vi "main 1.16 testing LR.vi"() -> ()   [LabVIEW 2015]
uses:
  subvi/PHOIBOS/DEFINITIONS/DEF_dev_state.ctl
  subvi/PHOIBOS/DEFINITIONS/DEF_dev_type.ctl
  <vilib>/Analysis/_algsub.llb/Real Vector Norm.vi
  <vilib>/Analysis/1siggen.llb/Ramp Pattern by Samples.vi
  <vilib>/DAQmx/create/channels.llb/DAQmx Create Channel (DI-Digital Input).vi
  <userlib>/caLab/Private/Put_DBL_PV.vi
  <vilib>/Utility/file.llb/Write Delimited Spreadsheet (string).vi
  <vilib>/Utility/file.llb/Read Delimited Spreadsheet (string).vi
  <vilib>/Utility/file.llb/Write Delimited Spreadsheet (DBL).vi
  <userlib>/caLab/Private/Get_PV.vi
  subvi/Newport ESP301/Newport ESP301.lvlib
  subvi/sp_manip.llb/sp_manip_lib.lvlib
  subvi/sp_manip.llb/tcp_gateway.lvlib
  <vilib>/Analysis/NI_AALBase.lvlib
  <vilib>/Analysis/NI_AALPro.lvlib
  subvi/ZaberTSeries/ZaberTSeries.lvlib
panel:
  out "Pics L":i32=200
  out "Waveform Chart":dbl(graph)
  out "G2 X":cluster{dbl[], "Ramp Pattern":dbl[]}(graph)
  in  "reset every n pics":bool=TRUE
  in  "pics2avg":i32=50
  in  "abort acq.":bool
  out "G2 Y":cluster{dbl[], "Ramp Pattern":dbl[]}(graph)
  out "ETA":timestamp=timestamp(3655133644.4615793 s since 1904-01-01) format="%<%H:%M:%S>T"
  out "acq. imgs":i32=200
  out "snap_prog":dbl(slide)=1.0 scale=0.0..1.0
  in  "BasePath":path=path "X:/trARPES/PESData"
  in  "cam_liveavg":bool=TRUE caption="live average"
  out "cam_fps":dbl=19.774122625512067 caption="FPS" format="%.1g"
  out "sideimg":dbl[][](graph)
  out "RunNumber":u16=3067
  out "sum":dbl format="%#.2g"
  out "max":dbl
  out "mainimg":dbl[][](graph)
  out "ESP_con?":bool=TRUE caption="ESP301"
  out "phoib_con?":bool caption="PHOIBOS"
  out "manip_con?":bool=TRUE caption="manipulator"
  out "cam_con?":bool caption="camera"
  in  "main_close":bool
  in  "Tab Control":enum32{"live", "1D scan", "devices"}(tab)
  out "Readback":dbl=304.0
  out "In Range":bool=TRUE
  in  "setpoint_set":bool
  in  "Setpoint":dbl=302.0
  out "TB":dbl=302.67
  out "TA":dbl=303.83
  in  "phoib_I_10s":dbl
  out "phoib_I_10":dbl caption="Mesh Back"
  in  "mirr_go":bool
  in  "ESP_opent0file":bool
  in  "mirr_rel":i32=1 caption="relative [steps]"
  in  "mirr_Y-":bool
  in  "mirr_Y+":bool
  in  "mirr_X+":bool
  in  "mirr_X-":bool
  in  "manip_deltas":dbl[](array[numeric])=[0.0, 0.0, 5.0, 0.0, 0.0, 0.0] caption="delta" format="%#.5g"
  in  "aq.mode":enum32{"Radio Selection 1", "Radio Selection 2"}(radio)=enum."Radio Selection 2"
  in  "dark avg":i32=100
  in  "cam_avgs":i32=200 caption="N"
  in  "ESP_delta":dbl caption="relative [mm]"
  in  "ESP_-":bool
  in  "ESP_+":bool
  in  "ESP_go":bool
  in  "ESP_dest_t":dbl=-1194159.4608093842 caption="[fs]"
  in  "ESP_dest":dbl=-324.0 caption="[mm]"
  in  "ESP_set_t0":bool
  in  "phoib_I_6s":dbl=3200.0
  in  "phoib_I_5s":dbl=1500.0
  in  "phoib_I_4s":dbl=4.558
  in  "phoib_I_3s":dbl=-10.0
  in  "phoib_I_2s":dbl=35.0
  in  "phoib_I_1s":dbl=21.0
  in  "phoib_standby":bool
  in  "phoib_set":bool
  out "phoib_I_6":dbl caption="Screen Voltage"
  out "phoib_I_5":dbl caption="Detctor Voltage"
  out "phoib_I_4":dbl caption="Work Function"
  out "phoib_I_3":dbl caption="Coil Current"
  out "phoib_I_2":dbl caption="Pass Energy"
  out "phoib_I_1":dbl caption="Kinetic Energy"
  out "Saved Positions":string[][](table)=[["ertwertwert", "-2.299945", "-2.030214", "38.900024", "50.000762", "0.000887", "-97.998082"], ["uztgugt", "-14.999451", "-13.638894", "442.380066", "13.998380", "-1.893758", "-76.305838"], ["asdf", "-14.999451", "-13.638894", "442.380066", "13.998380", "-1.893758", "-76.305838"], ["test3", "-14.999451", "-13.638894", "441.380066", "13.998380", "-1.893758", "-76.305838"]]
  in  "Save Pos":bool
  in  "Load":bool
  in  "Delete":bool
  in  "ManipRel +":bool
  in  "ManipRel -":bool
  in  "Move Abs":bool
  in  "stop manip":bool
  in  "dest":dbl[](array[numeric])=[1.794011231344732, -4.007411134769244, 35.099853515625, 337.9843004481455, 2.0, 140.61656469713384] caption="destination" format="%#.5g"
  out "axis":string[](array[string])=["x", "y", "z", "polar", "tilt", "azimut"]
  out "pos":dbl[](array[numeric])=[1.794011231344732, -4.007411134769244, 35.099853515625, 337.9843004481455, 1.998632949125299, 140.61656469713384] caption="position" format="%.5f"
  in  "ana_mode":T1(ring)=enum."WideAngleMode"
  in  "ana_voltrange":enum16{"3.5kV", "1.5kV", "400V", "100V", "10V"}(ring)=enum."400V"
  out "ESP_pos":dbl=-325.0 caption="Position"
  out "ESP_delay":dbl=-1200830.742713347 caption="Delay"
  out "ESP_t0":dbl=-145.0 caption="Time Zero @"
  out "phoib_I_7":dbl caption="Conversion Voltage"
  in  "phoib_I_7s":dbl=-30.0
  in  "phoib_I_8s":dbl=0.0039
  in  "phoib_I_9s":dbl
  out "phoib_I_8":dbl caption="FD1"
  out "phoib_I_9":dbl caption="Mesh Front"
  in  "gain":bool
  in  "cam_exp":u32=50 caption="exposure [ms]"
  in  "binning":u16(ring)=2 items=["X 1", "X 2", "X 4", "X 8"]
  in  "cam_dark?":bool=TRUE caption="subtract dark?"
  in  "cam_dark":bool
  in  "cam_saveimg":bool
  in  "e-size":u8
  in  "lower threshold":i32=50
  in  "count?":bool
  in  "ROI Left":i32=1
  in  "ROI Right":i32=43
  in  "ROI Top":i32=1
  in  "ROI Bottom":i32=33
  out "moving?":bool[](array[boolean])
  out "mirr_posX":i32=60782 caption="X"
  out "mirr_posY":i32=121383 caption="Y"
  in  "mirr_dest":i32[](array[numeric])=[60782, 121383]
  in  "clear delay table":bool
  out "anglegraph":dbl[][](graph)=[[0.0, 0.0, 0.0, 0.0, 0.0, 0.0, 0.0, 0.0, 0.0, 0.0, 0.0, 0.0, 0.0, 0.0, 0.0, 0.0, 0.0, 0.0, 0.0, 0.0, 0.0, 0.0, 0.0, 0.0, 0.0, 0.0, 0.0, 307.98, 204.45, 0.0, 0.0, 0.0, 0.0, 0.0, 0.0, 0.0, 0.0, 0.0, 0.0, 0.0, 0.0, 0.0, 0.0, 0.0, 0.0, 0.0, 0.0, 0.0, 0.0, 0.0, 0.0, 0.0, 0.0, 0.0, 0.0, 0.0, 0.0, 0.0, 0.0, 0.0, 0.0, 0.0, 0.0, 0.0, 0.0, 0.0, 0.0, 0.0, 0.0, 0.0, 0.0, 0.0, 0.0, 0.0, 0.0, 0.0, 0.0, 0.0, 0.0, 0.0, 0.0, 0.0, 0.0, 0.0, 0.0, 0.0, 0.0, 0.0, 0.0, 0.0, 0.0, 0.0, 0.0, 0.0, 0.0, 0.0, 0.0, 0.0, 0.0, 0.0, 0.0, 0.0, 0.0, 0.0, 0.0, 0.0, 0.0, 0.0, 0.0, 0.0, 0.0, 0.0, 0.0, 0.0, 0.0, 0.0, 0.0, 0.0, 0.0, 0.0, 0.0, 0.0, 0.0, 0.0, 0.0, 0.0, 0.0, 0.0, 0.0, 0.0, 0.0, 0.0, 0.0, 0.0, 0.0, 0.0, 0.0, 0.0, 0.0, 0.0, 0.0, 0.0, 0.0, 0.0, 0.0, 0.0, 0.0, 0.0, 0.0, 0.0, 0.0, 0.0, 0.0, 0.0, 0.0, 0.0, 640.8800000000001, 550.45, 91.89, 0.0, 0.0, 0.0, 0.0, 0.0, 0.0, 0.0, 0.0, 0.0, 0.0, 0.0, 0.0, 0.0, 0.0, 0.0, 0.0, 69.94, 60.96, 0.0, 0.0, 0.0, 0.0, 0.0, 0.0, 0.0, 0.0, 0.0, 0.0, 0.0, 0.0, 0.0, 0.0, 0.0, 0.0, 0.0, 0.0, 0.0, 115.87, 235.84, 172.04999999999998, 0.0, 0.0, 0.0, 0.0, 0.0, 0.0, 0.0, 0.0, 0.0, 0.0, 0.0, 0.0, 0.0, 0.0, 0.0, 0.0, 0.0, 0.0, 0.0, 0.0, 0.0, 0.0, 0.0, 0.0, 0.0, 0.0, 0.0, 0.0, 0.0, 0.0, 0.0, 0.0, 0.0, 0.0, 0.0, 0.0, 0.0, 0.0, 0.0, 0.0, 0.0, 0.0, 0.0, 0.0, 0.0, 0.0, 0.0, 0.0, 0.0, 0.0, 0.0, 0.0, 0.0, 0.0, 0.0, 0.0, 0.0], [0.0, 0.0, 0.0, 0.0, 0.0, 0.0, 0.0, 0.0, 0.0, 0.0, 0.0, 0.0, 0.0, 0.0, 0.0, 0.0, 54.97, 1426.6399999999999, 1312.94, 180.81, 0.0, 0.0, 0.0, 0.0, 0.0, 0.0, 0.0, 465.48, 989.61, 293.56, 0.0, 0.0, 0.0, 0.0, 0.0, 0.0, 0.0, 0.0, 0.0, 0.0, 0.0, 0.0, 0.0, 0.0, 0.0, 0.0, 0.0, 0.0, 0.0, 0.0, 0.0, 0.0, 0.0, 0.0, 0.0, 0.0, 0.0, 0.0, 0.0, 331.78, 944.91, 463.28, 0.0, 0.0, 0.0, 0.0, 143.70999999999998, 402.81, 196.09, 0.0, 0.0, 0.0, 483.82, 433.7, 0.0, 0.0, 0.0, 0.0, 0.0, 0.0, 89.85, 513.2, 263.03999999999996, 0.0, 0.0, 0.0, 0.0, 0.0, 0.0, 0.0, 0.0, 104.84, 0.0, 226.86, 214.93, 235.13, 0.0, 0.0, 0.0, 0.0, 0.0, 0.0, 0.0, 0.0, 0.0, 0.0, 0.0, 0.0, 0.0, 0.0, 0.0, 0.0, 0.0, 0.0, 0.0, 0.0, 0.0, 0.0, 0.0, 0.0, 0.0, 0.0, 0.0, 0.0, 0.0, 0.0, 0.0, 0.0, 0.0, 0.0, 0.0, 0.0, 0.0, 0.0, 0.0, 0.0, 0.0, 0.0, 0.0, 380.83, 649.96, 229.04, 0.0, 0.0, 0.0, 276.21000000000004, 441.79999999999995, 228.29, 0.0, 0.0, 0.0, 0.0, 0.0, 0.0, 0.0, 0.0, 0.0, 0.0, 0.0, 0.0, 0.0, 0.0, 0.0, 0.0, 0.0, 0.0, 0.0, 0.0, 123.92000000000002, 1311.81, 1454.81, 600.87, 0.0, 0.0, 0.0, 0.0, 0.0, 0.0, 0.0, 0.0, 0.0, 0.0, 0.0, 0.0, 0.0, 0.0, 0.0, 0.0, 0.0, 0.0, 0.0, 0.0, 0.0, 0.0, 0.0, 0.0, 0.0, 0.0, 0.0, 0.0, 0.0, 0.0, 654.53, 894.22, 410.35, 0.0, 0.0, 0.0, 0.0, 0.0, 0.0, 0.0, 0.0, 0.0, 0.0, 0.0, 0.0, 0.0, 0.0, 0.0, 0.0, 0.0, 0.0, 0.0, 0.0, 0.0, 0.0, 0.0, 0.0, 0.0, 0.0, 0.0, 0.0, 0.0, 0.0, 0.0, 0.0, 0.0, 0.0, 0.0, 0.0, 0.0, 0.0, 0.0, 0.0, 0.0, 0.0, 0.0, 0.0, 0.0, 0.0, 0.0, 0.0, 0.0, 0.0, 0.0], [0.0, 0.0, 0.0, 0.0, 0.0, 0.0, 0.0, 0.0, 0.0, 0.0, 0.0, 0.0, 0.0, 0.0, 0.0, 0.0, 0.0, 0.0, 0.0, 0.0, 0.0, 0.0, 0.0, 0.0, 0.0, 0.0, 0.0, 0.0, 0.0, 125.9, 1017.51, 504.48, 0.0, 0.0, 0.0, 0.0, 0.0, 0.0, 0.0, 0.0, 0.0, 0.0, 0.0, 0.0, 0.0, 0.0, 0.0, 0.0, 0.0, 0.0, 0.0, 0.0, 0.0, 0.0, 0.0, 0.0, 0.0, 0.0, 0.0, 0.0, 0.0, 0.0, 0.0, 0.0, 0.0, 0.0, 0.0, 0.0, 0.0, 0.0, 0.0, 0.0, 109.81, 66.88, 0.0, 0.0, 733.48, 806.32, 342.43, 0.0, 0.0, 0.0, 0.0, 0.0, 0.0, 0.0, 0.0, 0.0, 0.0, 0.0, 0.0, 0.0, 0.0, 0.0, 0.0, 0.0, 0.0, 0.0, 0.0, 0.0, 0.0, 0.0, 0.0, 0.0, 0.0, 174.07999999999998, 275.74, 429.21, 301.15999999999997, 0.0, 0.0, 0.0, 0.0, 0.0, 0.0, 0.0, 0.0, 0.0, 0.0, 0.0, 0.0, 0.0, 0.0, 0.0, 0.0, 0.0, 0.0, 0.0, 0.0, 0.0, 0.0, 0.0, 0.0, 0.0, 0.0, 0.0, 0.0, 0.0, 0.0, 0.0, 0.0, 0.0, 0.0, 0.0, 0.0, 0.0, 0.0, 0.0, 0.0, 0.0, 0.0, 0.0, 0.0, 0.0, 0.0, 0.0, 0.0, 0.0, 0.0, 0.0, 0.0, 0.0, 0.0, 0.0, 0.0, 0.0, 0.0, 0.0, 0.0, 0.0, 0.0, 0.0, 0.0, 0.0, 0.0, 252.98000000000002, 303.56, 60.91, 52.9, 53.13, 0.0, 0.0, 0.0, 0.0, 0.0, 0.0, 0.0, 0.0, 0.0, 0.0, 0.0, 0.0, 0.0, 0.0, 0.0, 0.0, 0.0, 0.0, 0.0, 0.0, 0.0, 0.0, 0.0, 0.0, 0.0, 0.0, 0.0, 0.0, 0.0, 0.0, 0.0, 0.0, 0.0, 61.05, 350.49, 266.71000000000004, 0.0, 0.0, 0.0, 0.0, 0.0, 0.0, 0.0, 0.0, 0.0, 0.0, 0.0, 0.0, 0.0, 0.0, 0.0, 0.0, 0.0, 0.0, 0.0, 0.0, 0.0, 0.0, 0.0, 0.0, 0.0, 0.0, 0.0, 0.0, 0.0, 0.0, 0.0, 0.0, 0.0, 0.0, 0.0, 0.0, 0.0, 0.0, 0.0, 0.0]]
  out "intensitygraph":cluster{"Array":dbl[], "Intensity Chart":dbl[]}(graph)={"Array"=[302.0, 303.0, 304.0], "Intensity Chart"=[1937.88, 12704.590000000002, 4640.840000000001]}
  in  "scan_selector":enum32{"delay", "manip", "mirror", "T", "volt"}(tab)=enum."T"
  in  "scan_manip_setstart":bool
  in  "scan_manip_start":dbl[](array[numeric])=[1.794011231344732, -4.007411134769244, 35.099853515625, 337.9843004481455, 2.000390761745462, 140.61656469713384] caption="start position" format="%#.5g"
  in  "scan_manip_deltas":dbl[](array[numeric])=[0.0, 0.0, 0.0, 0.0, 1.0, 0.0] caption="direction vector\n(gets normed)" format="%#.5g"
  in  "scan_mirr_start":i32[](array[numeric])=[60782, 121383]
  in  "scan_mirr_deltas":i32[](array[numeric])=[1, 0] caption="direction vector\n(gets normed)"
  in  "scan_mirr_setstart":bool
  in  "wait addional":dbl caption="s"
  in  "Wait for T":bool=TRUE
  in  "scan_volt_parameter":string(combo)="Kinetic Energy"
  in  "meas_iter":i32=1 caption="Iterations"
  out "duration [HH:MM:SS]":dbl=32.361351013183594 format="%<%H:%M:%S>t"
  out "disk [MB]":dbl=1.6590000000000003
  out "RAM [MB]":dbl=1.6590000000000003
  out "total steps":i32=3
  out "measpoints":i32=3
  in  "load delay table":bool
  in  "scan_go":bool
  in  "waypoints":string[][](table)=[["302", "1"], ["304", ""], ["", ""]]
  in  "stop after step":bool
  out "scan":dbl(slide)=1.0 scale=0.0..1.0
  out "iteration":dbl(slide)=1.0 scale=0.0..1.0
  out "current scan":i32=3
  out "current iteration":i32=1
  in  "time/step [s]":dbl=10.787117004394531
  in  "stop after iteration":bool
  out "energygraph":dbl[][](graph)=[[0.0, 0.0, 0.0, 64.28999999999999, 120.06, 0.0, 0.0, 0.0, 0.0, 0.0, 0.0, 0.0, 0.0, 0.0, 0.0, 0.0, 0.0, 0.0, 0.0, 0.0, 0.0, 0.0, 0.0, 0.0, 0.0, 0.0, 0.0, 0.0, 0.0, 0.0, 0.0, 0.0, 0.0, 0.0, 0.0, 0.0, 0.0, 0.0, 0.0, 0.0, 0.0, 0.0, 0.0, 0.0, 0.0, 0.0, 0.0, 0.0, 0.0, 384.53999999999996, 1103.3799999999999, 448.21000000000004, 0.0, 0.0, 0.0, 0.0, 0.0, 0.0, 0.0, 0.0, 0.0, 0.0, 0.0, 0.0, 0.0, 0.0, 0.0, 0.0, 0.0, 120.82, 0.0, 261.04, 195.1, 253.87, 199.70999999999998, 127.75, 87.50999999999999, 0.0, 52.54, 0.0, 0.0, 51.78, 55.73, 0.0, 0.0, 0.0, 0.0, 0.0, 0.0, 0.0, 0.0, 0.0, 0.0, 0.0, 0.0, 0.0, 0.0, 0.0, 0.0, 0.0, 0.0, 0.0, 0.0, 0.0, 0.0, 0.0, 0.0, 0.0, 0.0, 0.0, 0.0, 0.0, 0.0, 332.90999999999997, 1106.25, 934.74, 0.0, 156.76, 62.65, 0.0, 0.0, 0.0, 0.0, 0.0, 0.0, 54.62, 0.0, 0.0, 0.0, 0.0, 0.0, 0.0, 0.0, 0.0, 0.0, 0.0, 0.0, 0.0, 0.0, 0.0, 0.0, 0.0, 0.0, 0.0, 65.85, 165.75, 0.0, 0.0, 0.0, 0.0, 0.0, 0.0, 0.0, 0.0, 0.0, 0.0, 0.0, 0.0, 0.0, 0.0, 0.0, 0.0, 0.0, 266.63, 591.5, 261.64, 0.0, 391.9, 527.29, 82.87, 123.75, 286.74, 151.72, 0.0, 0.0, 0.0, 0.0, 0.0, 0.0, 0.0, 0.0, 0.0, 0.0, 0.0, 0.0, 0.0, 0.0, 0.0, 0.0, 0.0, 0.0, 0.0, 396.37, 721.0900000000001, 353.5, 83.97999999999999, 104.77000000000001, 0.0, 57.83, 60.98, 182.28, 128.78, 0.0, 0.0, 0.0, 465.25, 624.3399999999999, 348.62, 0.0, 0.0, 0.0, 0.0, 0.0, 0.0, 0.0, 0.0, 0.0, 0.0, 0.0, 0.0, 119.7, 217.91, 120.56, 0.0, 0.0, 0.0, 0.0, 0.0, 0.0, 0.0, 58.89, 0.0, 0.0, 0.0, 202.23999999999998, 149.79000000000002, 0.0, 117.82, 212.51999999999998, 534.74, 421.98, 50.97, 0.0, 0.0, 0.0, 0.0, 362.15999999999997, 656.04, 265.02, 0.0, 0.0, 0.0, 0.0, 0.0, 0.0, 0.0, 0.0, 0.0, 0.0, 0.0, 0.0, 0.0, 0.0, 0.0, 0.0, 0.0, 0.0, 0.0, 0.0, 0.0, 0.0, 0.0, 0.0, 0.0, 0.0, 0.0, 0.0, 0.0, 0.0, 0.0, 0.0, 0.0, 0.0, 0.0, 0.0, 0.0, 0.0, 0.0, 0.0, 0.0, 0.0, 0.0, 0.0, 0.0, 0.0, 0.0, 0.0, 0.0, 0.0, 0.0, 0.0, 0.0, 0.0, 0.0, 0.0, 0.0, 0.0, 0.0, 0.0, 0.0, 0.0, 0.0, 0.0, 237.67999999999998, 286.08, 130.9, 0.0, 0.0, 0.0, 0.0, 0.0, 0.0, 0.0, 0.0, 0.0, 0.0, 0.0, 0.0, 0.0, 0.0, 0.0, 0.0, 0.0, 0.0, 0.0, 0.0, 0.0, 0.0, 0.0, 0.0, 0.0, 0.0, 0.0, 0.0], [0.0, 0.0, 0.0, 0.0, 0.0, 0.0, 0.0, 0.0, 0.0, 0.0, 0.0, 0.0, 0.0, 0.0, 0.0, 0.0, 0.0, 485.13, 1279.2, 234.71, 0.0, 0.0, 0.0, 0.0, 0.0, 0.0, 0.0, 0.0, 0.0, 0.0, 0.0, 0.0, 50.5, 654.4200000000001, 511.98, 0.0, 0.0, 0.0, 0.0, 0.0, 0.0, 0.0, 0.0, 0.0, 0.0, 0.0, 0.0, 0.0, 0.0, 0.0, 0.0, 0.0, 0.0, 0.0, 0.0, 0.0, 0.0, 0.0, 63.72, 693.84, 574.54, 0.0, 0.0, 0.0, 68.68, 1054.28, 1010.9499999999999, 0.0, 0.0, 0.0, 0.0, 0.0, 0.0, 0.0, 0.0, 0.0, 0.0, 0.0, 56.57, 971.76, 1333.73, 330.0, 0.0, 0.0, 0.0, 0.0, 0.0, 349.33000000000004, 292.7, 0.0, 0.0, 0.0, 0.0, 0.0, 0.0, 82.77000000000001, 1059.23, 1069.87, 156.47, 0.0, 0.0, 0.0, 0.0, 293.91, 333.47, 551.4, 493.64, 73.72999999999999, 0.0, 0.0, 0.0, 0.0, 0.0, 0.0, 0.0, 0.0, 0.0, 0.0, 0.0, 0.0, 0.0, 0.0, 286.01, 543.0699999999999, 251.94, 0.0, 0.0, 0.0, 0.0, 0.0, 233.63, 968.4799999999999, 771.53, 109.94, 0.0, 123.07, 499.72999999999996, 431.4, 0.0, 0.0, 60.85, 69.5, 0.0, 0.0, 0.0, 0.0, 0.0, 0.0, 0.0, 0.0, 0.0, 0.0, 0.0, 0.0, 0.0, 0.0, 52.01, 0.0, 0.0, 0.0, 0.0, 0.0, 0.0, 0.0, 0.0, 0.0, 0.0, 0.0, 0.0, 0.0, 0.0, 0.0, 0.0, 0.0, 0.0, 0.0, 0.0, 0.0, 0.0, 0.0, 0.0, 0.0, 0.0, 0.0, 0.0, 0.0, 0.0, 0.0, 0.0, 0.0, 52.95, 478.8, 870.47, 572.83, 61.67, 268.19, 1143.4, 1804.2599999999998, 1145.6100000000001, 739.22, 904.59, 1109.3000000000002, 1233.6599999999999, 212.92, 0.0, 0.0, 105.95, 448.76000000000005, 1306.3500000000001, 1005.5900000000001, 68.8, 0.0, 57.94, 0.0, 0.0, 0.0, 0.0, 0.0, 0.0, 0.0, 0.0, 0.0, 0.0, 0.0, 0.0, 0.0, 0.0, 0.0, 0.0, 0.0, 0.0, 0.0, 0.0, 0.0, 0.0, 0.0, 0.0, 159.01, 520.94, 925.5600000000001, 1641.53, 2261.26, 1259.83, 0.0, 0.0, 0.0, 0.0, 0.0, 0.0, 136.69, 398.81, 382.02, 0.0, 0.0, 0.0, 0.0, 0.0, 0.0, 421.01, 1376.5800000000002, 1425.75, 268.07, 0.0, 345.84000000000003, 396.77, 0.0, 0.0, 0.0, 0.0, 0.0, 216.93, 727.65, 830.9, 774.2299999999999, 839.3900000000001, 309.97, 0.0, 0.0, 0.0, 0.0, 0.0, 0.0, 0.0, 100.57, 459.66, 305.86, 0.0, 0.0, 0.0, 0.0, 0.0, 0.0, 0.0, 0.0, 0.0, 0.0, 0.0, 0.0, 0.0, 0.0, 0.0, 0.0, 0.0, 0.0, 0.0, 0.0, 0.0, 0.0, 0.0, 0.0, 0.0, 64.97999999999999, 379.62, 337.15999999999997, 83.6, 463.66, 399.03999999999996, 0.0, 0.0, 0.0, 0.0, 0.0, 0.0, 0.0, 0.0, 0.0, 0.0, 0.0, 0.0, 0.0, 0.0, 0.0, 0.0, 0.0, 0.0, 0.0, 0.0, 0.0, 0.0, 0.0, 0.0, 0.0, 0.0, 0.0], [0.0, 0.0, 0.0, 0.0, 0.0, 0.0, 0.0, 0.0, 0.0, 0.0, 0.0, 0.0, 0.0, 0.0, 0.0, 165.83, 124.99, 78.27000000000001, 0.0, 0.0, 0.0, 765.77, 1457.88, 293.67, 0.0, 0.0, 0.0, 0.0, 0.0, 0.0, 0.0, 0.0, 0.0, 0.0, 0.0, 0.0, 0.0, 0.0, 0.0, 0.0, 0.0, 0.0, 0.0, 0.0, 0.0, 0.0, 0.0, 0.0, 0.0, 85.5, 116.32, 0.0, 0.0, 0.0, 0.0, 0.0, 0.0, 0.0, 0.0, 0.0, 0.0, 0.0, 0.0, 0.0, 0.0, 0.0, 0.0, 0.0, 179.01, 123.78999999999999, 64.69, 0.0, 433.57000000000005, 1457.15, 661.49, 0.0, 0.0, 0.0, 0.0, 0.0, 0.0, 171.38, 497.28999999999996, 835.47, 1797.0300000000002, 1202.25, 169.95, 0.0, 0.0, 0.0, 0.0, 383.74, 496.08, 196.89999999999998, 0.0, 0.0, 0.0, 0.0, 719.08, 1717.5100000000002, 1360.8, 163.65, 118.56, 798.75, 610.32, 0.0, 0.0, 0.0, 0.0, 73.12, 51.75, 0.0, 0.0, 0.0, 0.0, 0.0, 0.0, 0.0, 0.0, 0.0, 0.0, 0.0, 233.35000000000002, 1128.3, 1138.8400000000001, 207.43, 0.0, 0.0, 50.52, 0.0, 0.0, 0.0, 0.0, 0.0, 0.0, 0.0, 0.0, 0.0, 0.0, 0.0, 0.0, 0.0, 0.0, 0.0, 0.0, 0.0, 0.0, 0.0, 0.0, 0.0, 0.0, 122.82, 66.93, 184.87, 606.35, 1065.2, 616.33, 82.97, 0.0, 0.0, 0.0, 0.0, 0.0, 0.0, 0.0, 0.0, 0.0, 0.0, 0.0, 210.77, 369.49, 0.0, 0.0, 0.0, 0.0, 0.0, 0.0, 0.0, 0.0, 0.0, 0.0, 0.0, 0.0, 0.0, 0.0, 0.0, 0.0, 0.0, 0.0, 61.71, 492.70000000000005, 501.67999999999995, 50.9, 0.0, 0.0, 0.0, 0.0, 0.0, 0.0, 0.0, 0.0, 0.0, 0.0, 0.0, 0.0, 0.0, 0.0, 0.0, 0.0, 0.0, 0.0, 0.0, 0.0, 0.0, 0.0, 0.0, 0.0, 0.0, 0.0, 0.0, 0.0, 0.0, 0.0, 0.0, 0.0, 0.0, 0.0, 0.0, 0.0, 0.0, 0.0, 0.0, 0.0, 0.0, 0.0, 0.0, 0.0, 0.0, 0.0, 0.0, 0.0, 0.0, 0.0, 0.0, 0.0, 0.0, 0.0, 0.0, 0.0, 0.0, 0.0, 0.0, 0.0, 0.0, 0.0, 0.0, 0.0, 0.0, 0.0, 0.0, 0.0, 0.0, 0.0, 0.0, 0.0, 0.0, 0.0, 0.0, 0.0, 0.0, 191.69, 347.02, 262.31, 325.89, 168.79, 0.0, 0.0, 52.9, 53.13, 0.0, 0.0, 0.0, 0.0, 0.0, 0.0, 0.0, 0.0, 0.0, 0.0, 0.0, 0.0, 0.0, 0.0, 0.0, 0.0, 0.0, 0.0, 0.0, 0.0, 0.0, 0.0, 0.0, 0.0, 0.0, 0.0, 327.12, 491.83000000000004, 242.02999999999997, 0.0, 0.0, 0.0, 0.0, 0.0, 0.0, 0.0, 676.6, 975.77, 229.86, 0.0, 144.15, 151.75, 0.0, 0.0, 0.0, 0.0, 0.0, 0.0, 0.0, 0.0, 0.0, 0.0, 0.0, 0.0, 0.0, 0.0, 0.0, 0.0, 0.0, 0.0, 0.0, 0.0, 0.0, 0.0, 0.0]]
  in  "LS310  EPICS Heater":string="trARPES:Carving:HT-RNG"
  in  "LS310  EPICS SP":string="trARPES:Carving:TEMP"
  in  "LS310  EPICS chanel B":string="trARPES:Carving:TEMP-B"
  in  "mm/s":dbl
  in  "Set Speed to":bool
  in  "ESP Axis waveplate":i32=2 min=1 max=3
  in  "mirr_init":bool
  in  "mirr_release":bool
  in  "mirr_Y#":u8=2
  in  "manip_init":bool
  in  "manip_release":bool
  in  "phoib_init":bool
  in  "phoib_release":bool
  in  "ESP_init":bool
  in  "ESP_release":bool
  in  "ESP301 VISA":refnum<visa-resource-name>="COM4"
  in  "board number":i32
  in  "cam_init":bool
  in  "cam_release":bool
  out "cam_error":errorcluster
  out "phoib_error":errorcluster
  out "state":T2 items=["Off"=-1, "Standby"=0, "On"=1]
  in  "ESP Axis delay":i32=3 min=1 max=3
  out "error out":errorcluster={"status"=FALSE, "code"=1073676418, "source"="VISA Close in Newport ESP301.lvlib:Close.vi->main 1.16 testing LR.vi"}
  out "error out 2":errorcluster={"status"=TRUE, "code"=1, "source"="TCP Write in sp_manip_lib.lvlib:sp_manip_disconnect.vi->main 1.16 testing LR.vi"}
  out "mirr_Error":errorcluster={"status"=FALSE, "code"=1073676418, "source"="VISA Close in ZaberTSeries.lvlib:Close.vi->main 1.16 testing LR.vi"}
  in  "mirr_VISA":refnum<visa-resource-name>="COM7"
  in  "mirr_X#":u8=1
  in  "Operating mode\nHP & QE / HS & DiCam Pro":u32=1
  in  "Frame trigger \n(High Performance and QE only)":u16
  in  "LS310  EPICS chanel A":string="trARPES:Carving:TEMP_RBV"
  in  "Status EPICS chanel":string="trARPES:Carving:TEMP-STAT"
  # "camera"
  # "analyzer"
  # "manipulator"
  # "temperature"
  # "aquisition"
  # "delay stage"
  # "mirror"
  # "Position"
  # "Destination"
  # "- no settings -"
  # "waypoints are absolute values"
  # "X\nY\nZ\npolar\ntilt\nazimut"
  # "waypoint \"0\" is start position"
  # "X\nY"
  # "waypoint \"0\" is start position"
  # "waypoints are absolute values"
  # "camera"
  # "phoibos"
  # "ESP301"
  # "manipulator"
  # "mirror"
  # "0 = sequential\n1 = simultaneous"
  # "0 = internal\n1 = external rising\n2 = external falling"
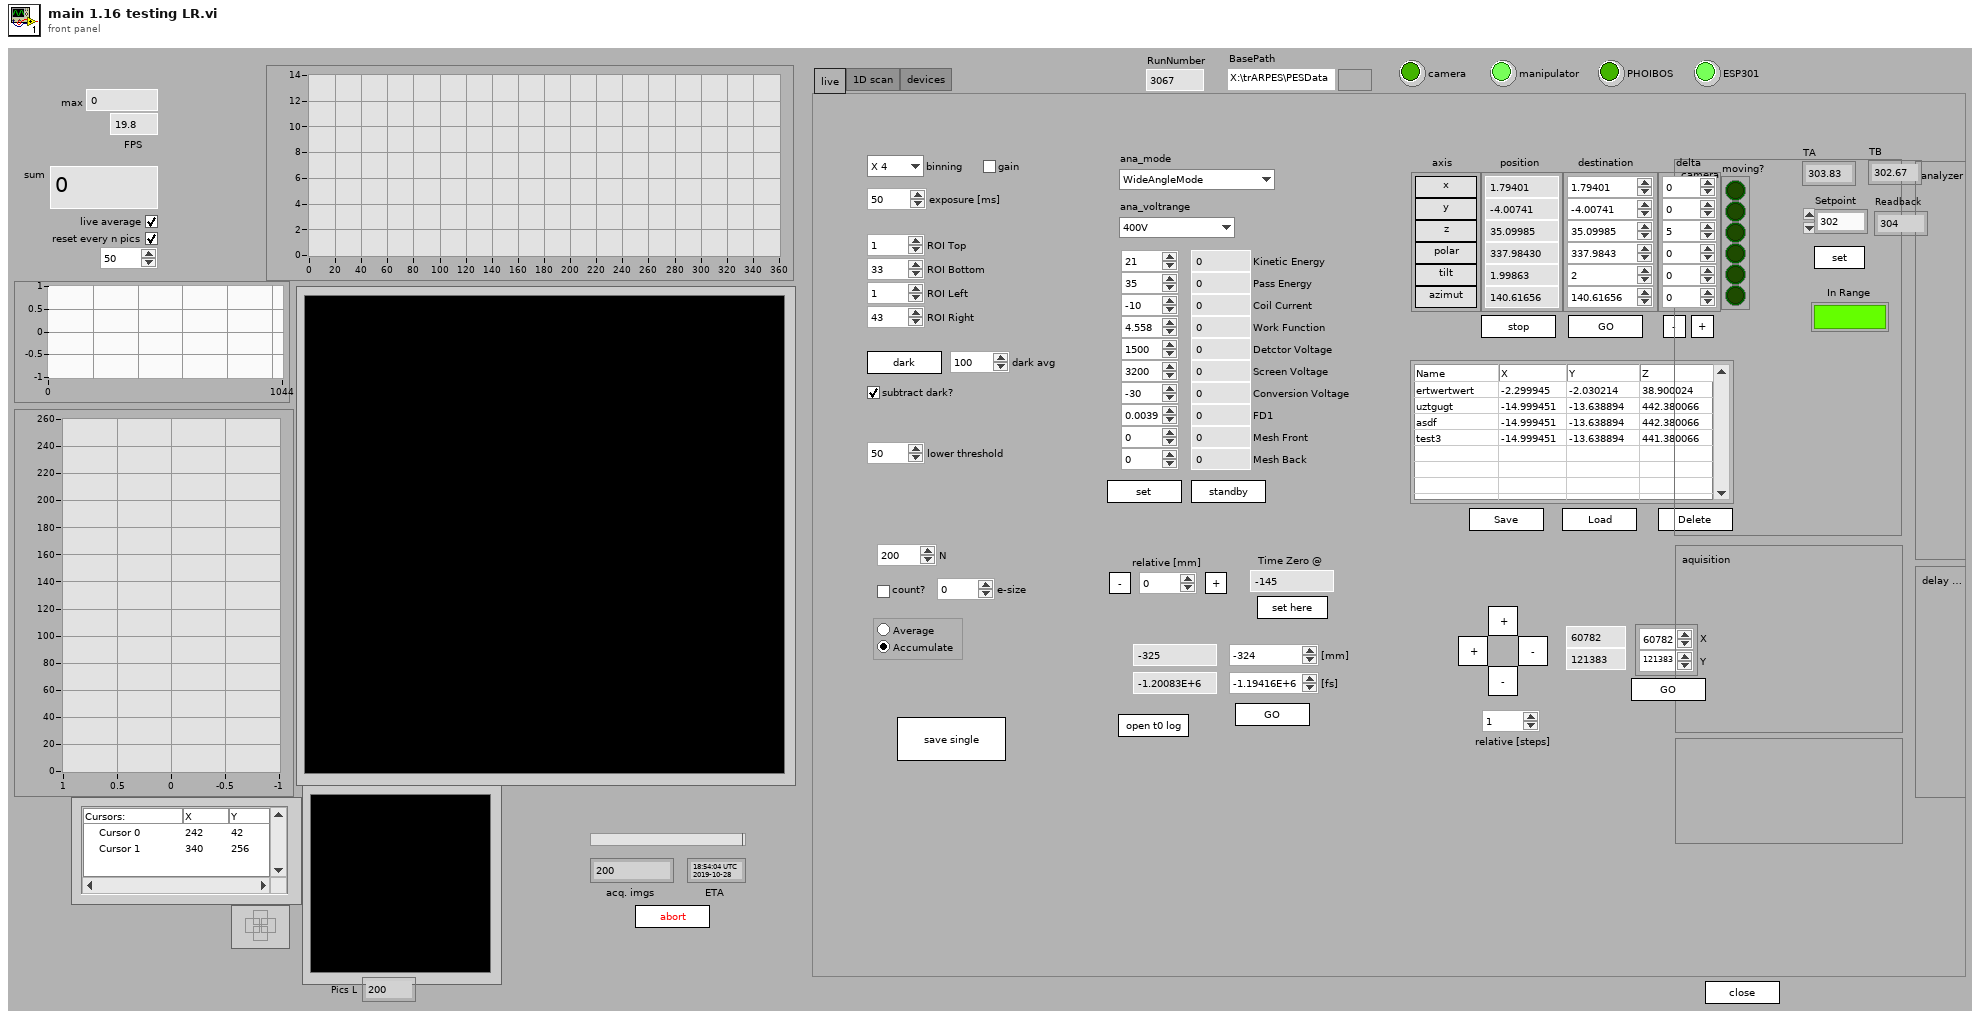
[diagram p1: front panel]
types:
  T1 = enum16{"HighMagnification", "MediumMagnification", "LowMagnification", "HighAngularDispersion", "MediumAngularDispersion", "LowAngularDispersion", "WideAngleMode", "LargeArea", "MediumArea", "SmallArea", "HighMagnification2", "SmallArea2"}
  T2 = typedef "DEF_dev_state.ctl" = i32
  T3 = cluster{"queue out":refnum<queue>, "queue out":refnum<queue>, "queue out":refnum<queue>, "queue out":refnum<queue>, "queue out":refnum<queue>, "queue out":refnum<queue>}
  T4 = typedef "LVCursorListTypeDef.ctl" = cluster{"Name":string, "Color":u32, "Style":u8, "Point Style":u8, "Name Visible":bool, "Allow Drag":bool, "Cursor Mode":u32, "Plot":i32, "Index":i32, "Position":cluster{"X":dbl, "Y":dbl}, "X Scale":u32, "Y Scale":u32, "Watch Plots":i32[], "Watch All Plots":bool, "Plot Area":i32, "Label Offset":cluster{"X":dbl, "Y":dbl}}[]
  T5 = cluster{"Camera type":u32, "Operating mode\nHP & QE / HS & DiCam Pro ":u32, "Frame trigger \n(High Performance and QE only)":u16, "Sequence trigger":u16, "Low Light\n(QE only)":bool, "Gain":bool, "Horzontal\nbinning":u16, "Vertical\nbinning ":u16, "ROI Left":i32, "ROI Right":i32, "ROI Top":i32, "ROI Bottom":i32}
  T6 = cluster{"Name":string, "Color":u32, "Style":u8, "Point Style":u8, "Name Visible":bool, "Allow Drag":bool, "Cursor Mode":u32, "Plot":i32, "Index":i32, "Position":cluster{"X":dbl, "Y":dbl}, "X Scale":u32, "Y Scale":u32, "Watch Plots":i32[], "Watch All Plots":bool, "Plot Area":i32, "Label Offset":cluster{"X":dbl, "Y":dbl}}
  T7 = cluster{"mirr_X#":u8, "Command":u8, dbl, "Response Count":i32}
  T8 = cluster{"mirr_Y#":u8, "Command":u8, dbl, "Response Count":i32}
  T9 = cluster{i32, "Command":u8, i32, "Response Count":i32}
  T10 = cluster{"Axis_Name":string, "Axis_Type":string, "Axis_Position":dbl, "continous":bool, "moving":bool}[]
  T11 = typedef "DEF_dev_type.ctl" = enum32{"devA (analyzer)", "devD (detector)"}
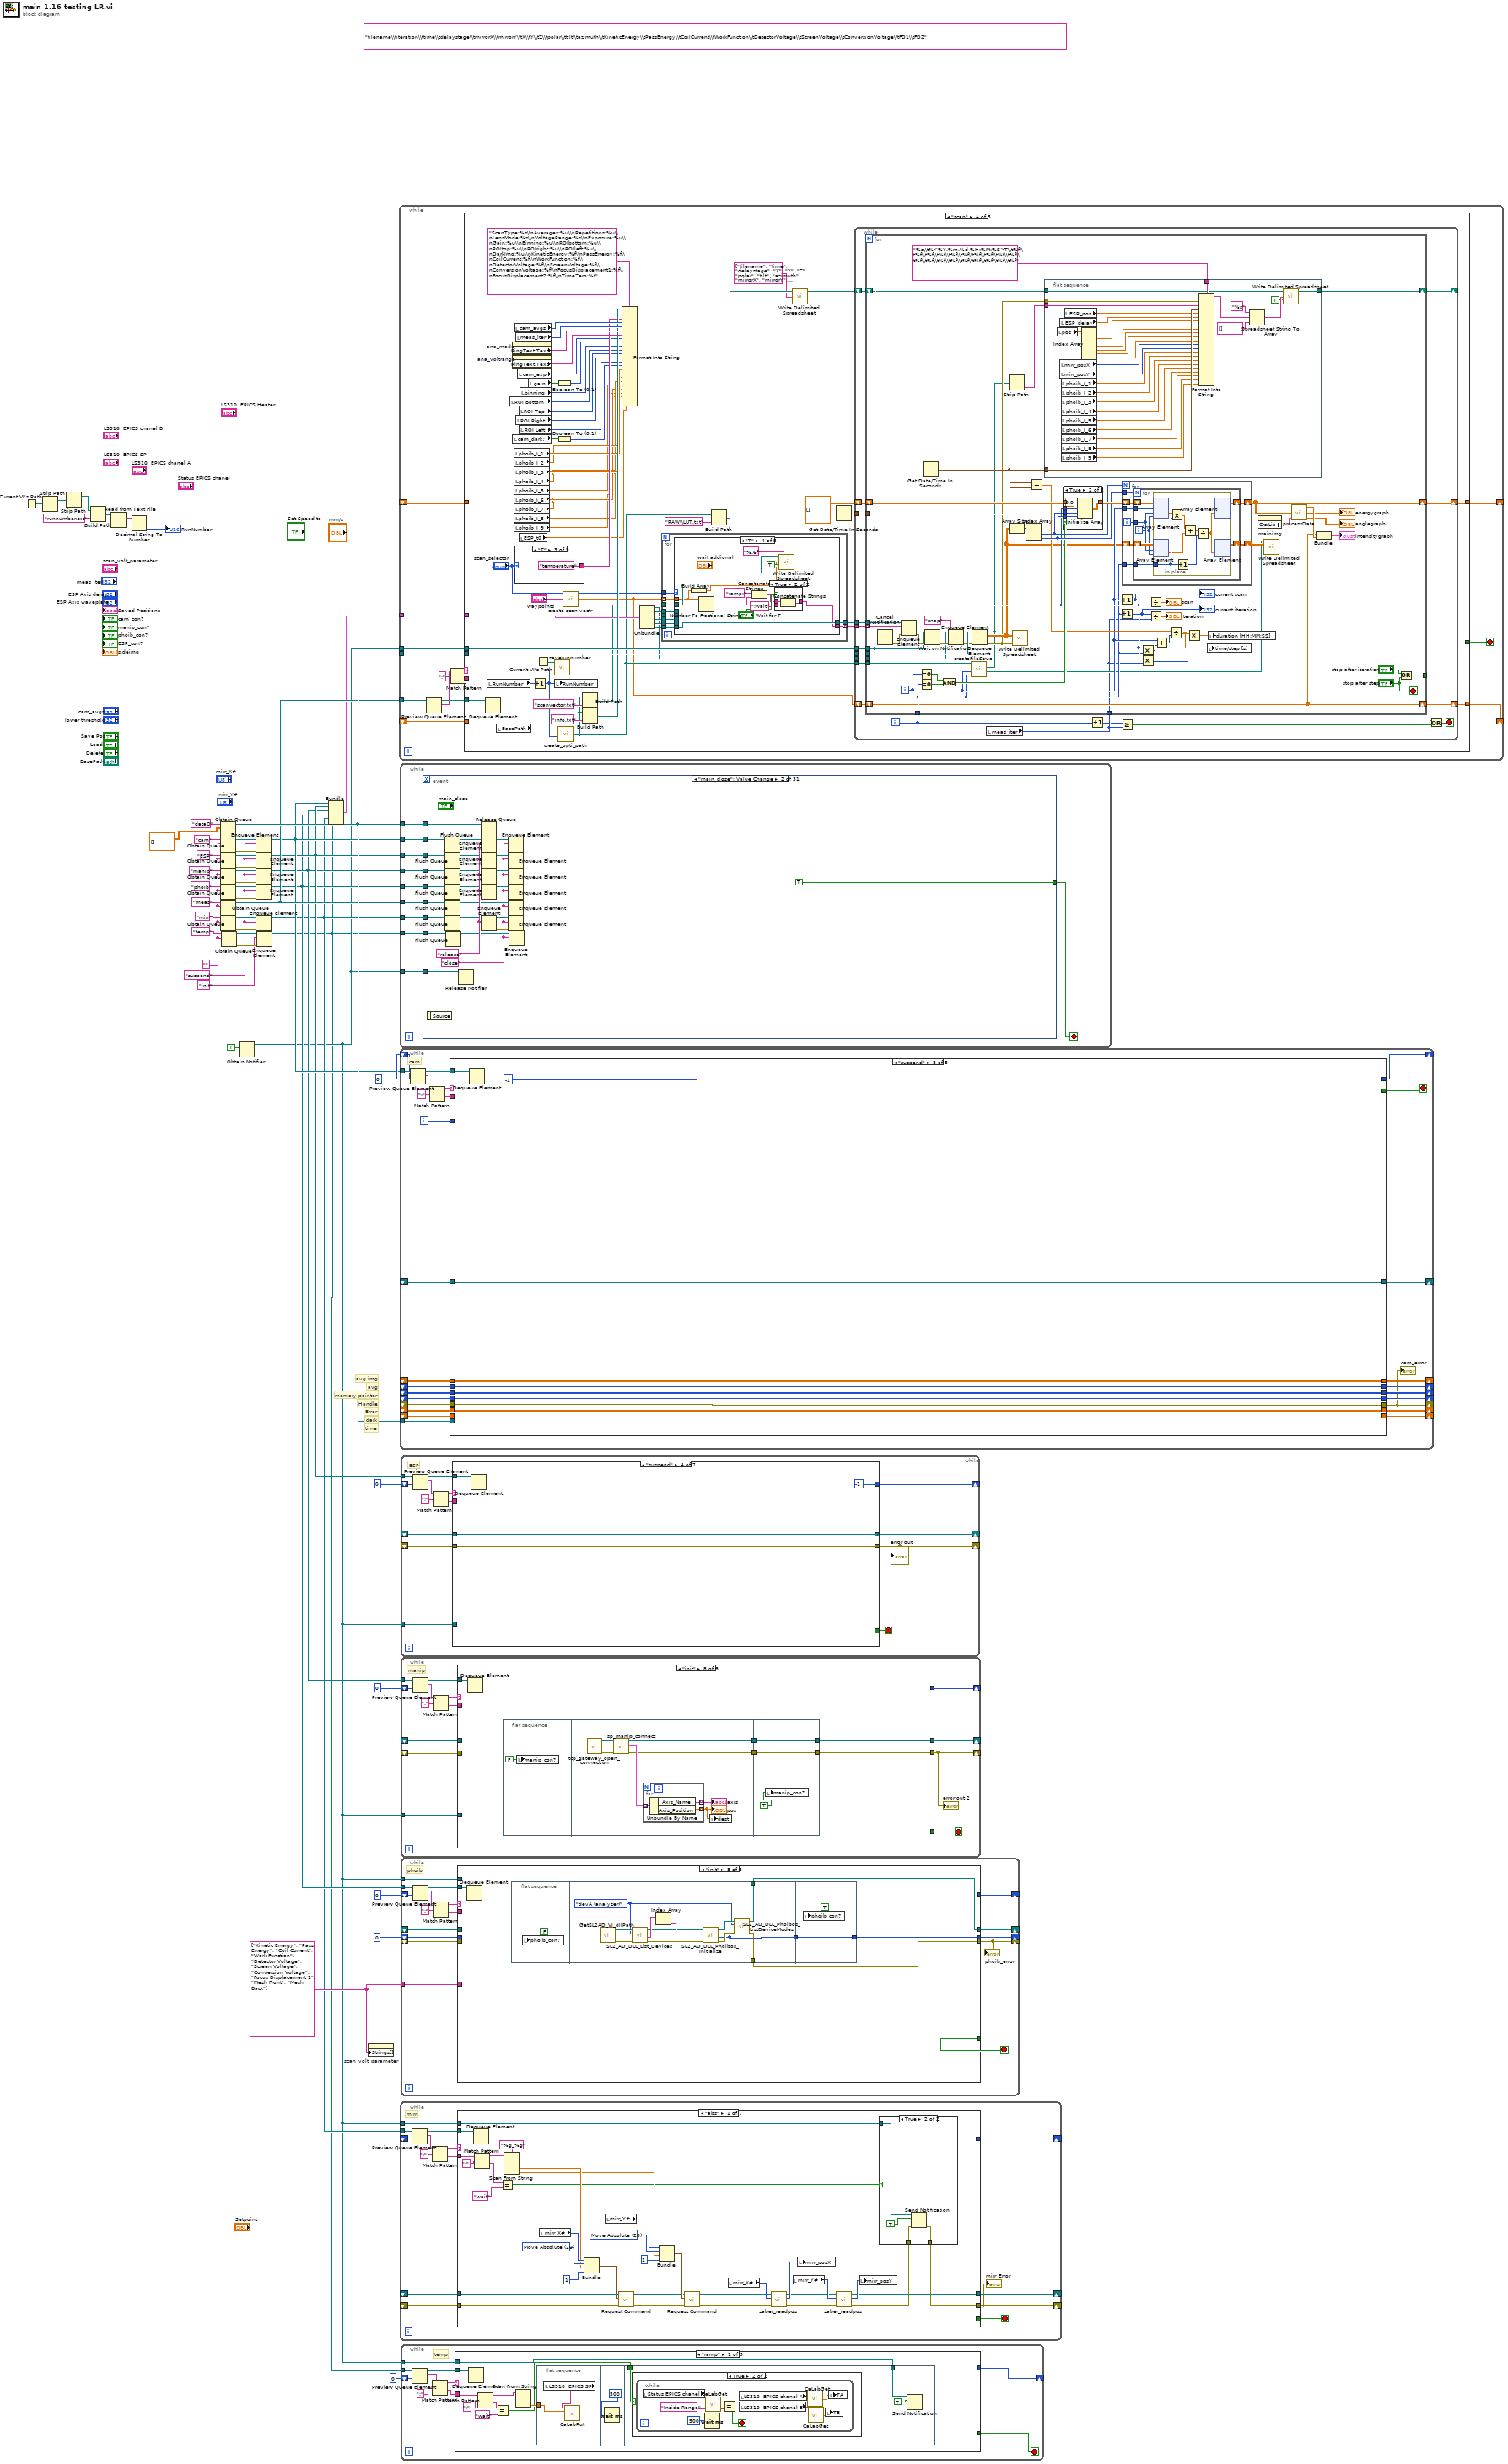
[diagram p0: block diagram]
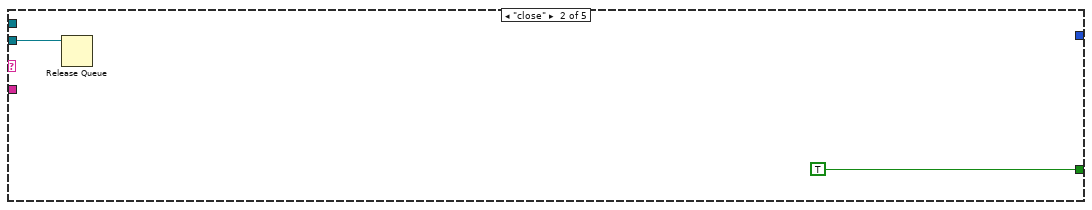
[diagram p3: hidden frame]
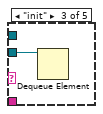
[diagram p4: hidden frame]
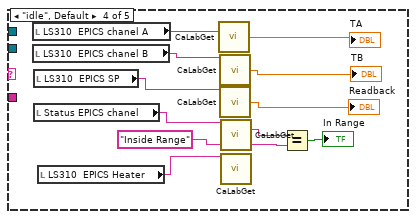
[diagram p5: hidden frame]
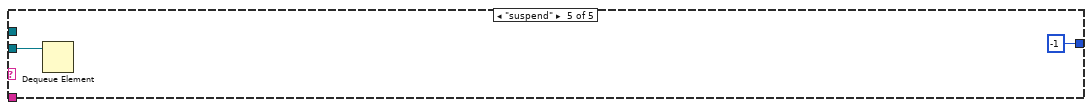
[diagram p6: hidden frame]
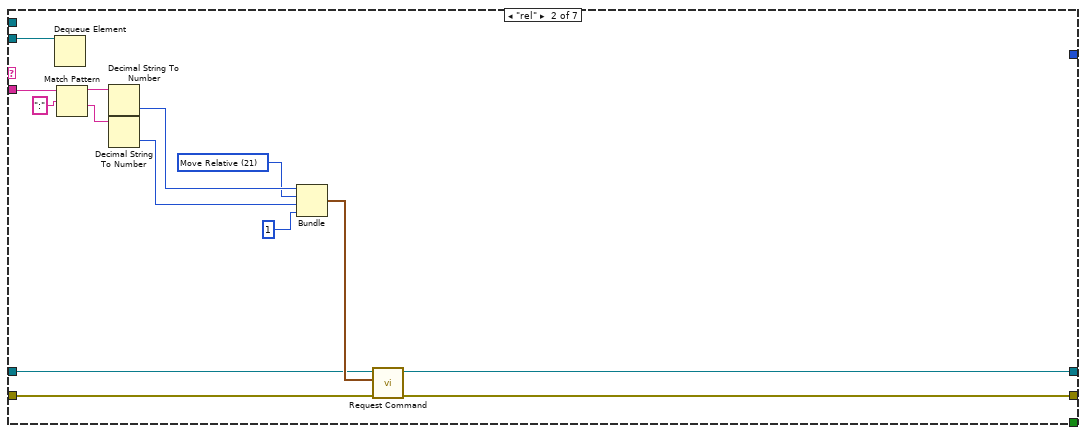
[diagram p8: hidden frame]
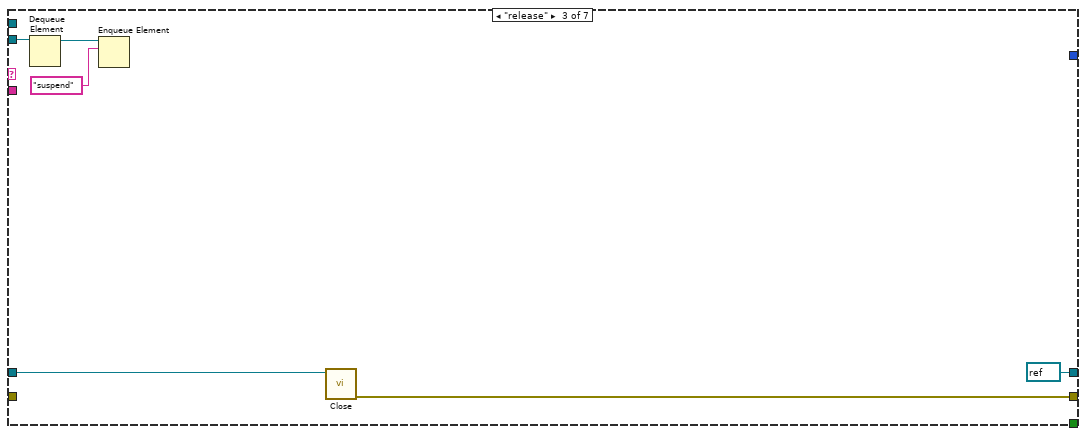
[diagram p9: hidden frame]
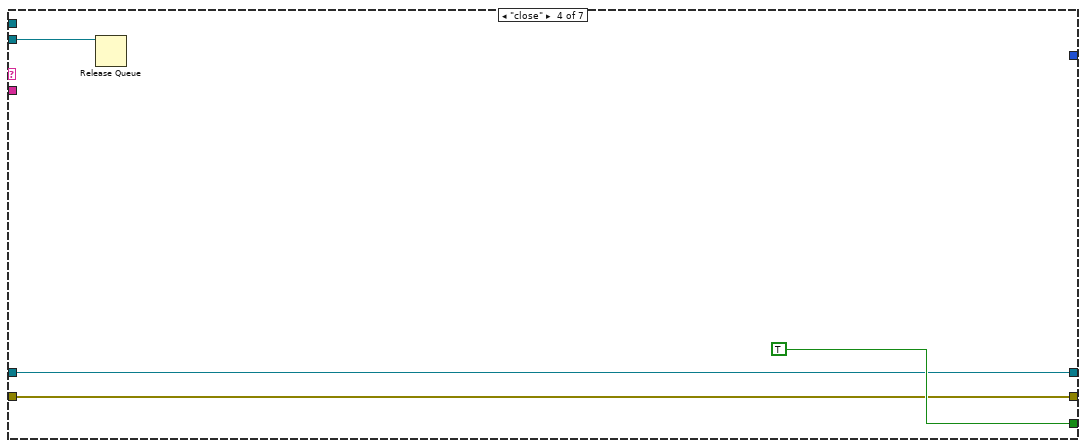
[diagram p10: hidden frame]
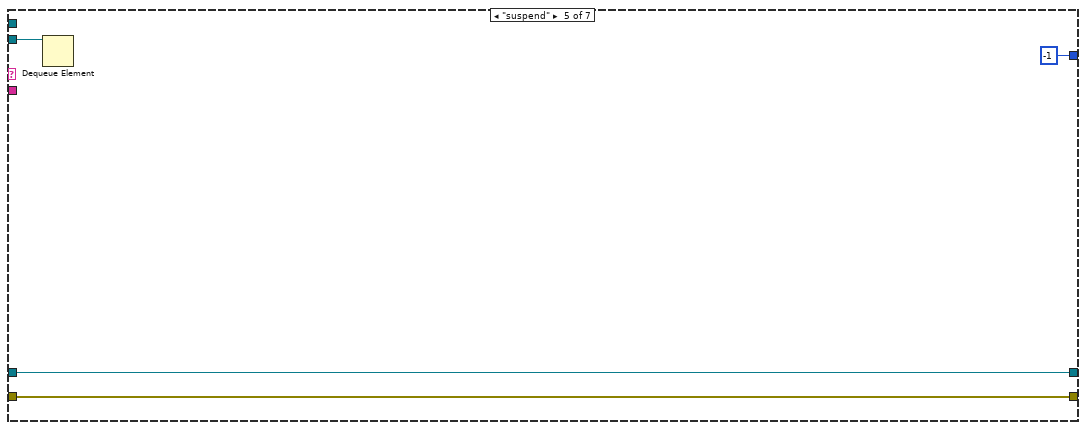
[diagram p11: hidden frame]
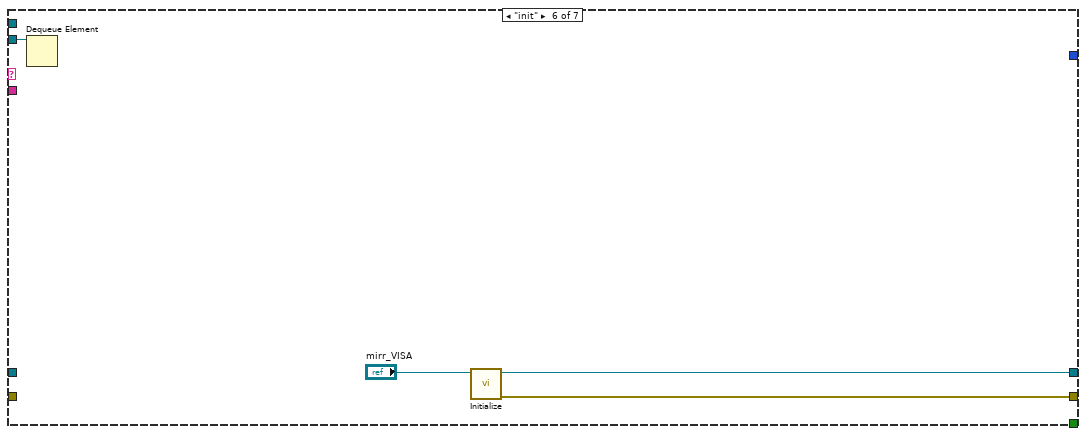
[diagram p12: hidden frame]
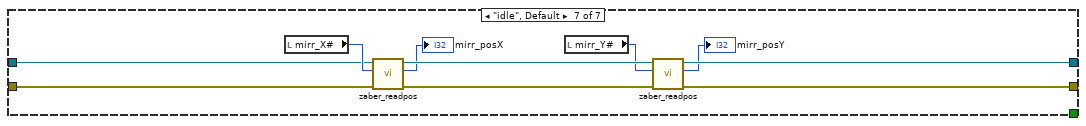
[diagram p13: hidden frame]
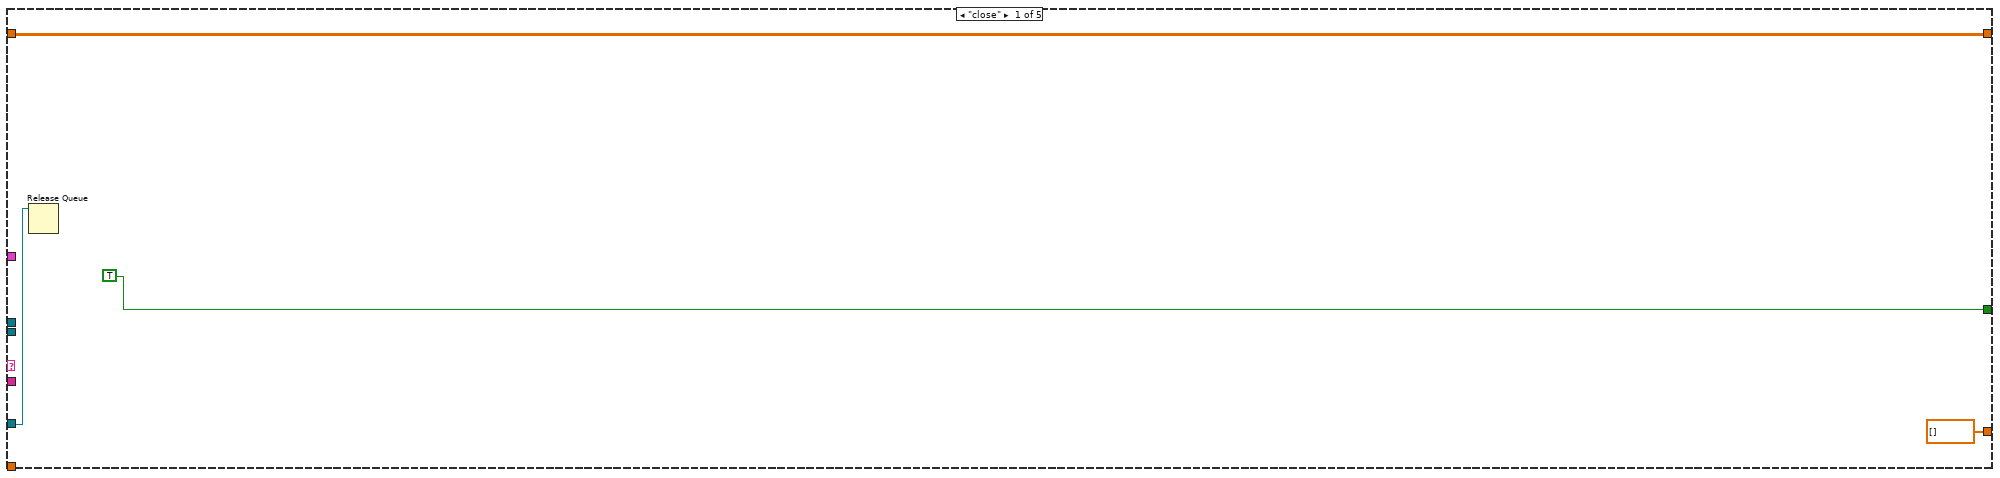
[diagram p14: hidden frame]
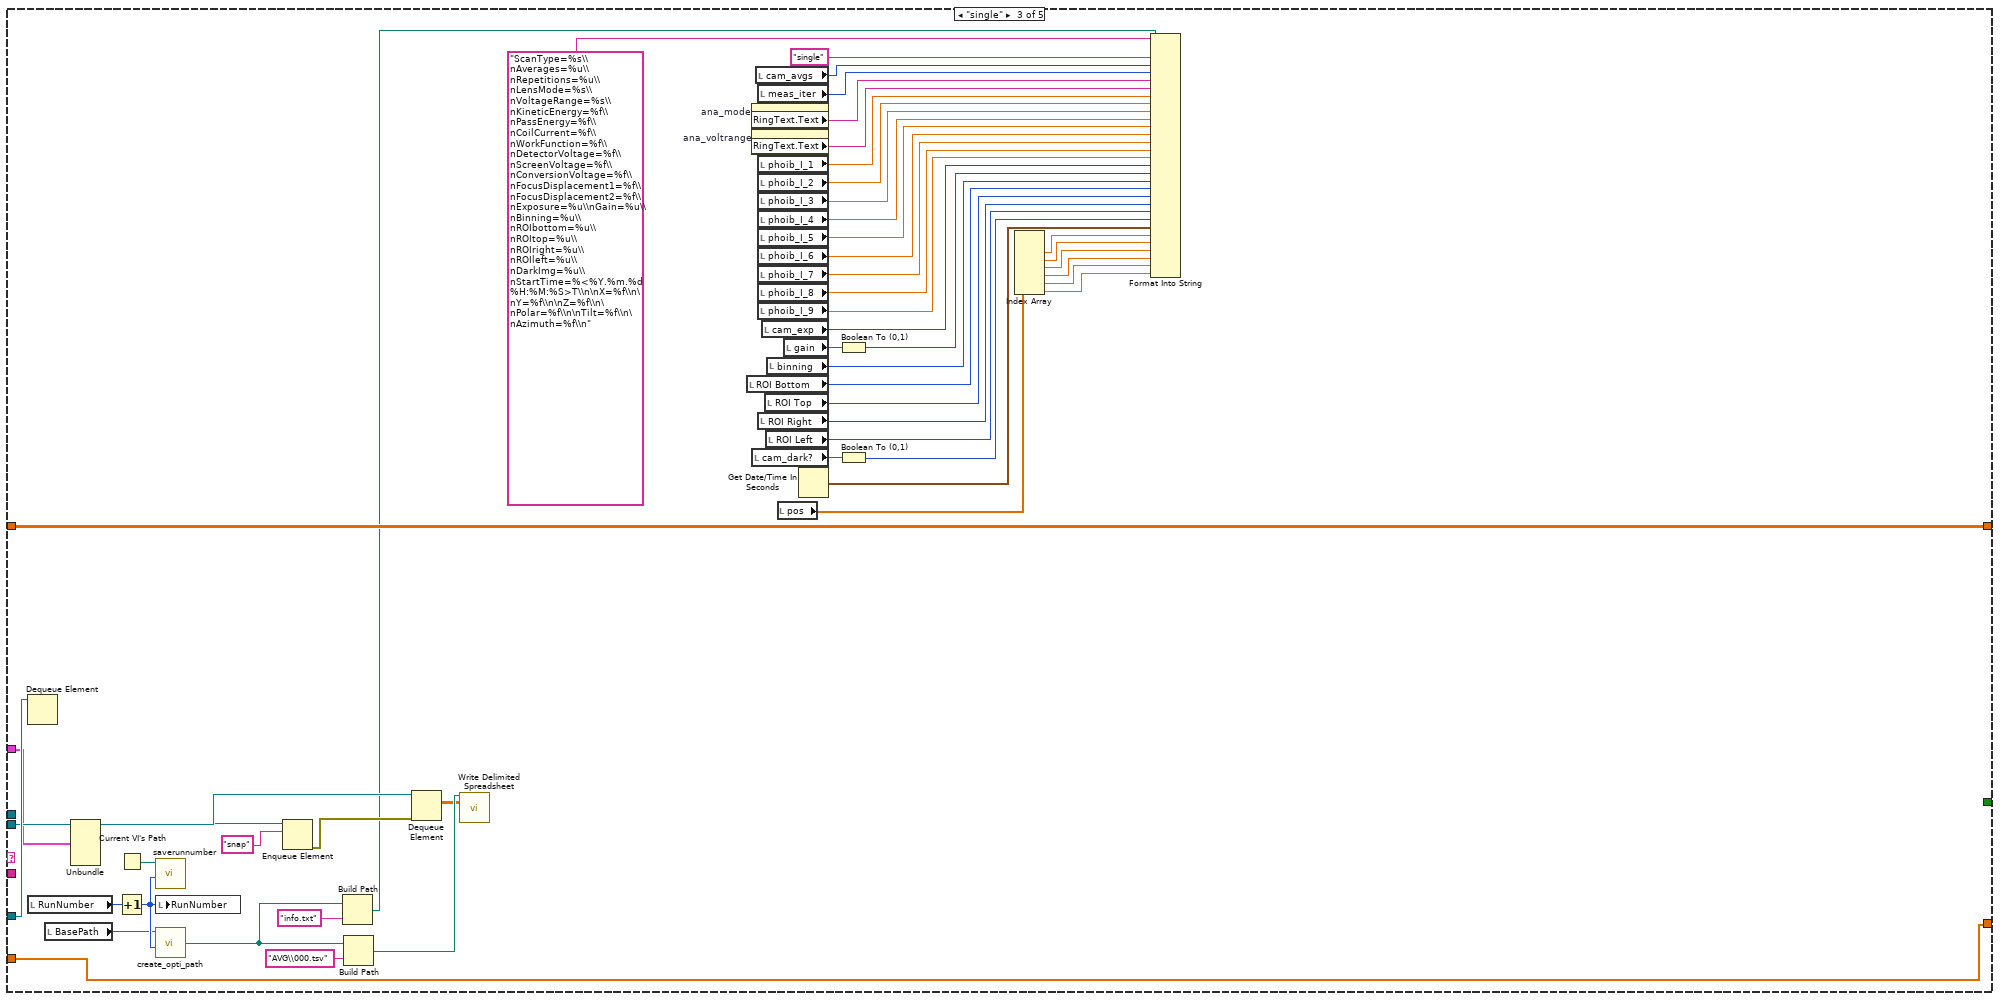
[diagram p16: hidden frame]
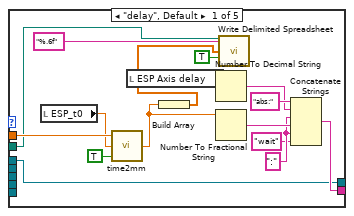
[diagram p18: hidden frame]
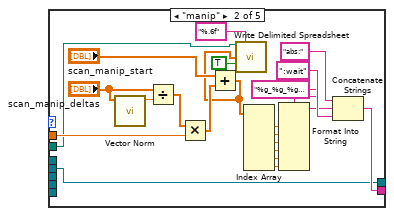
[diagram p19: hidden frame]
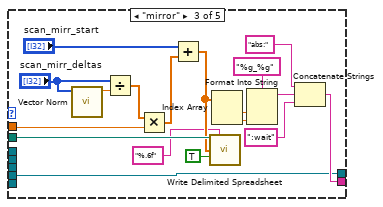
[diagram p20: hidden frame]
diagram:
  (unwired) "filename\\titeration\\ttime\\tdelaystage\\tmirrorX\\tmirrorY\\tX\\tY\\tZ\\tpolar\\ttilt\\tazimuth\\tKineticEnergy\\tPassEnergy\\tCoilCurrent\\tWorkFunction\\tDetectorVoltage\\tScreenVoltage\\tConversionVoltage\\tFD1\\tFD2"
  w15 = string[] ["Kinetic Energy", "Pass Energy", "Coil Current", "Work Function", "Detector Voltage", "Screen Voltage", "Conversion Voltage", "Focus Displacement 1", "Mesh Front", "Mesh Back"]
  w3 = "suspend" ("name (unnamed)")
  w8 = "" ("name (unnamed)")
  # "avg img"
  # "avg"
  # "time"
  # "dark"
  # "Error"
  # "Handle"
  # "memory pointer"
  n1 = Current VI's Path() -> (path=w23:path)
  n2 = Strip Path(path=w23) -> (stripped path=w27:path)  [unwired: 1 out]
  n3 = Strip Path(path=w27) -> (stripped path=w28:path)  [unwired: 1 out]
  n4 = Build Path(base path=w28, name or relative path="runnumber.txt") -> (appended path=w25:path)
  n5 = Read from Text File(file (use dialog)=w25) -> (text=w26:string)  [unwired: 3 in, 3 out]
  n6 = Decimal String To Number(string=w26) -> (number=→"RunNumber":i32)  [unwired: 2 in, 1 out]
  n7 = Obtain Queue(name (unnamed)="dataQ", element data type=dbl[][] []) -> (queue out=w29:refnum<queue>)  [unwired: 3 in, 2 out]
  n8 = Obtain Queue(name (unnamed)="cam", element data type=w8) -> (queue out=w48:refnum<queue>, error out=w47:errorcluster)  [unwired: 3 in, 1 out]
  n9 = Obtain Queue(name (unnamed)="ESP", element data type=w8) -> (queue out=w45:refnum<queue>, error out=w46:errorcluster)  [unwired: 3 in, 1 out]
  n10 = Obtain Queue(name (unnamed)="manip", element data type=w8) -> (queue out=w42:refnum<queue>, error out=w41:errorcluster)  [unwired: 3 in, 1 out]
  n11 = Obtain Queue(name (unnamed)="phoib", element data type=w8) -> (queue out=w39:refnum<queue>, error out=w40:errorcluster)  [unwired: 3 in, 1 out]
  n12 = Obtain Queue(name (unnamed)="meas", element data type=w8) -> (queue out=w22:refnum<queue>)  [unwired: 3 in, 2 out]
  n13 = Obtain Queue(name (unnamed)="mirr", element data type=w8) -> (queue out=w13:refnum<queue>, error out=w12:errorcluster)  [unwired: 3 in, 1 out]
  n14 = Obtain Queue(name (unnamed)="temp", element data type=w8) -> (queue out=w7:refnum<queue>, error out=w6:errorcluster)  [unwired: 3 in, 1 out]
  n15 = Obtain Notifier(notification data type=TRUE) -> (notifier out=w5:refnum<notifier>)  [unwired: 3 in, 2 out]
  n16 = Enqueue Element(queue=w48, element=w3, error in (no error)=w47) -> (queue out=w20:refnum<queue>)  [unwired: 1 in, 2 out]
  n17 = Enqueue Element(queue=w45, element=w3, error in (no error)=w46) -> (queue out=w19:refnum<queue>)  [unwired: 1 in, 2 out]
  n18 = Enqueue Element(queue=w42, element=w3, error in (no error)=w41) -> (queue out=w18:refnum<queue>)  [unwired: 1 in, 2 out]
  n19 = Enqueue Element(queue=w39, element=w3, error in (no error)=w40) -> (queue out=w17:refnum<queue>)  [unwired: 1 in, 2 out]
  n20 = Enqueue Element(queue=w13, element=w3, error in (no error)=w12) -> (queue out=w10:refnum<queue>)  [unwired: 1 in, 2 out]
  n21 = Enqueue Element(queue=w7, element="init" ("name (unnamed)"), error in (no error)=w6) -> (queue out=w1:refnum<queue>)  [unwired: 1 in, 2 out]
  n22 = Bundle("queue out"=w20, "queue out"=w19, "queue out"=w18, "queue out"=w17, "queue out"=w10, "queue out"=w1) -> (w21:T3)  [unwired: 1 in]
  n23 = property on="scan_volt_parameter" class="CmbBox"("Strings[]"=w15) -> ()  [unwired: 2 in, 2 out]
  n24 = while {
    tunnel: w29 -> [w63]
    tunnel: w22 -> [w60]
    tunnel: w21 -> [w56]
    shift-right: [w54] -> _
    shift-left: _ -> [w53]
    tunnel: w5 -> [w52]
    shift-right: [w51] -> _
    shift-left: _ -> [w50]
    stop <- w55 stop-if-true
    n25 = Preview Queue Element(queue=w60) -> (queue out=w57:refnum<queue>, element=w62:string)  [unwired: 2 in, 2 out]
    n26 = Match Pattern(string=w62, regular expression=":") -> (before substring=w59:string, after substring=w58:string)  [unwired: 1 in, 2 out]
    n27 = case shown="\"scan\"" w59 {
      tunnel: w63 -> [_ _ w119 w172 _]
      tunnel: w58 -> [_ _ _ _ _]
      tunnel: w57 -> [w67 _ w120 w168 w410]
      tunnel: [TRUE _ _ _ _] -> w55
      tunnel: w56 -> [_ _ w107 w148 _]
      tunnel: [w65 w69 w105 w170 w416] -> w54
      tunnel: w53 -> [w65 w69 w105 _ w416]
      tunnel: w52 -> [_ _ _ w169 _]
      tunnel: [dbl[] [] ("Array") w68 w77 w134 w412] -> w51
      tunnel: w50 -> [_ w68 w77 _ w412]
      frame "close" {
        n28 = Release Queue(queue=w67) -> ()  [unwired: 2 in, 3 out]
      }
      frame "idle", Default {
      }
      frame "single" {
        n29 = Dequeue Element(queue=w120) -> ()  [unwired: 2 in, 4 out]
        n30 = local read "RunNumber"() -> (w114:u16)
        n31 = local read "BasePath"() -> (w115:path)
        n32 = Unbundle(w107) -> ("queue out"=w106:refnum<queue>)  [unwired: 5 out]
        n33 = Increment(x=w114) -> (x+1=w116:u16)
        n34 = Current VI's Path() -> (path=w113:path)
        n35 = call "saverunnumber.vi"("RunNumber"=w116, "VI path"=w113) -> ()  [unwired: 10 in]
        n36 = local write "RunNumber"(w116) -> ()
        n37 = call "create_opti_path.vi"("RunNumber"=w116, "base path"=w115) -> ("Path"=w109:path)  [unwired: 2 in]
        n38 = Enqueue Element(queue=w106, element="snap" ("string")) -> (error out=w117:errorcluster)  [unwired: 2 in, 2 out]
        n39 = Build Path(base path=w109, name or relative path="info.txt") -> (appended path=w78:path)
        n40 = Build Path(base path=w109, name or relative path="AVG\\000.tsv") -> (appended path=w111:path)
        n41 = Dequeue Element(queue=w119, error in (no error)=w117) -> (element=w108:dbl[][])  [unwired: 1 in, 3 out]
        n42 = call-poly <vilib>:"Write Delimited Spreadsheet.vi"("file path (dialog if empty)"=w111, "2D data"=w108) -> ()  [unwired: 12 in, 2 out]
        n43 = local read "ROI Bottom"() -> (w85:i32)
        n44 = property on="ana_mode" class="Enum (strict)"() -> ("RingText.Text"=w100:string)  [unwired: 2 in, 2 out]
        n45 = property on="ana_voltrange" class="Enum (strict)"() -> ("RingText.Text"=w99:string)  [unwired: 2 in, 2 out]
        n46 = local read "cam_dark?"() -> (w81:bool)
        n47 = local read "cam_avgs"() -> (w102:i32)
        n48 = local read "meas_iter"() -> (w101:i32)
        n49 = local read "phoib_I_1"() -> (w98:dbl)
        n50 = local read "phoib_I_2"() -> (w97:dbl)
        n51 = local read "phoib_I_3"() -> (w96:dbl)
        n52 = local read "phoib_I_4"() -> (w95:dbl)
        n53 = local read "phoib_I_5"() -> (w94:dbl)
        n54 = local read "phoib_I_6"() -> (w93:dbl)
        n55 = local read "phoib_I_7"() -> (w92:dbl)
        n56 = local read "phoib_I_8"() -> (w91:dbl)
        n57 = local read "phoib_I_9"() -> (w90:dbl)
        n58 = local read "ROI Right"() -> (w83:i32)
        n59 = local read "cam_exp"() -> (w89:u32)
        n60 = local read "ROI Top"() -> (w84:i32)
        n61 = local read "ROI Left"() -> (w82:i32)
        n62 = local read "binning"() -> (w86:u16)
        n63 = local read "pos"() -> (w76:dbl[])
        n64 = local read "gain"() -> (w88:bool)
        n65 = Get Date/Time In Seconds() -> (seconds since 1Jan1904=w79:timestamp)
        n66 = Boolean To (0,1)(Boolean=w88) -> (0, 1=w87:i16)
        n67 = Boolean To (0,1)(Boolean=w81) -> (0, 1=w80:i16)
        n68 = Index Array(array=w76) -> (element #1=w75:dbl, element #2=w74:dbl, element #3=w73:dbl, element #4=w72:dbl, element #5=w71:dbl, element #6=w70:dbl)  [unwired: 6 in]
        n69 = Format Into String(format string="ScanType=%s\\nAverages=%u\\nRepetitions=%u\\nLensMode=%s\\nVoltageRange=%s\\nKineticEnergy=%f\\nPassEnergy=%f\\nCoilCurrent=%f\\nWorkFunction=%f\\nDetectorVoltage=%f\\nScreenVoltage=%f\\nConversionVoltage=%f\\nFocusDisplacement1=%f\\nFocusDisplacement2=%f\\nExposure=%u\\nGain=%u\\nBinning=%u\\nROIbottom=%u\\nROItop=%u\\nROIright=%u\\nROIleft=%u\\nDarkImg=%u\\nStartTime=%<%Y.%m.%d %H:%M:%S>T\\n\nX=%f\\n\nY=%f\\n\nZ=%f\\n\nPolar=%f\\n\nTilt=%f\\n\nAzimuth=%f\\n", initial string=w78, "single" ("input 1"), w102, w101, w100, w99, w98, w97, w96, w95, w94, w93, w92, w91, w90, w89, w87, w86, w85, w84, w83, w82, w80, w79, w75, w74, w73, w72, w71, w70) -> ()  [unwired: 1 in, 2 out]
      }
      frame "scan" {
        n70 = Dequeue Element(queue=w168) -> ()  [unwired: 2 in, 4 out]
        n71 = local read "RunNumber"() -> (w176:u16)
        n72 = local read "BasePath"() -> (w177:path)
        n73 = local read "ROI Bottom"() -> (w154:i32)
        n74 = property on="ana_mode" class="Enum (strict)"() -> ("RingText.Text"=w163:string)  [unwired: 2 in, 2 out]
        n75 = property on="ana_voltrange" class="Enum (strict)"() -> ("RingText.Text"=w162:string)  [unwired: 2 in, 2 out]
        n76 = local read "cam_dark?"() -> (w160:bool)
        n77 = local read "phoib_I_1"() -> (w132:dbl)
        n78 = local read "phoib_I_2"() -> (w131:dbl)
        n79 = local read "phoib_I_3"() -> (w130:dbl)
        n80 = local read "phoib_I_4"() -> (w129:dbl)
        n81 = local read "phoib_I_5"() -> (w128:dbl)
        n82 = local read "phoib_I_6"() -> (w127:dbl)
        n83 = local read "phoib_I_7"() -> (w126:dbl)
        n84 = local read "phoib_I_8"() -> (w125:dbl)
        n85 = local read "phoib_I_9"() -> (w124:dbl)
        n86 = local read "cam_avgs"() -> (w165:i32)
        n87 = case shown="\"T\"" "scan_selector" {
          tunnel: ["delay" ("input 1") "manipulator" ("input 1") "temperature" "mirror" ("input 1") "voltage" ("input 1")] -> w158
          frame "delay", Default {
          }
          frame "manip" {
          }
          frame "T" {
          }
          frame "mirror" {
          }
          frame "volt" {
          }
        }
        n88 = local read "meas_iter"() -> (w164:i32)
        n89 = local read "ROI Right"() -> (w152:i32)
        n90 = local read "cam_exp"() -> (w157:u32)
        n91 = local read "ROI Top"() -> (w153:i32)
        n92 = local read "ESP_t0"() -> (w123:dbl)
        n93 = local read "ROI Left"() -> (w151:i32)
        n94 = local read "binning"() -> (w155:u16)
        n95 = local read "gain"() -> (w161:bool)
        n96 = Increment(x=w176) -> (x+1=w178:u16)
        n97 = Current VI's Path() -> (path=w175:path)
        n98 = call "saverunnumber.vi"("RunNumber"=w178, "VI path"=w175) -> ()  [unwired: 10 in]
        n99 = local write "RunNumber"(w178) -> ()
        n100 = Boolean To (0,1)(Boolean=w161) -> (0, 1=w156:i16)
        n101 = Boolean To (0,1)(Boolean=w160) -> (0, 1=w150:i16)
        n102 = call "create_opti_path.vi"("RunNumber"=w178, "base path"=w177) -> ("Path"=w139:path)  [unwired: 2 in]
        n103 = call "create scan vectr.vi"("Table Control"="waypoints") -> ("Array"=w133:dbl[])
        n104 = Build Path(base path=w139, name or relative path="scanvector.txt") -> (appended path=w122:path)
        n105 = Build Path(base path=w139, name or relative path="info.txt") -> (appended path=w159:path)
        n106 = Format Into String(format string="ScanType:%s\\nAverages:%u\\nRepetitions:%u\\nLensMode:%s\\nVoltageRange:%s\\nExposure:%u\\nGain:%u\\nBinning:%u\\nROIbottom:%u\\nROItop:%u\\nROIright:%u\\nROIleft:%u\\nDarkImg:%u\\nKineticEnergy:%f\\nPassEnergy:%f\\nCoilCurrent:%f\\nWorkFunction:%f\\nDetectorVoltage:%f\\nScreenVoltage:%f\\nConversionVoltage:%f\\nFocusDisplacement1:%f\\nFocusDisplacement2:%f\\nTimeZero:%f", initial string=w159, w158, w165, w164, w163, w162, w157, w156, w155, w154, w153, w152, w151, w150, w132, w131, w130, w129, w128, w127, w126, w125, w124, w123) -> ()  [unwired: 1 in, 2 out]
        n107 = Unbundle(w148) -> ("queue out"=w140:refnum<queue>, "queue out"=w147:refnum<queue>, "queue out"=w146:refnum<queue>, "queue out"=w145:refnum<queue>, "queue out"=w144:refnum<queue>, "queue out"=w121:refnum<queue>)
        n108 = for {
          tunnel: w133 -> [w321] mode=indexing
          tunnel: [w320] -> w141 mode=indexing
          tunnel: [w319] -> w142
          tunnel: w147 -> [w318]
          tunnel: w146 -> [w317]
          tunnel: w145 -> [w316]
          tunnel: w144 -> [w315]
          tunnel: "scan_selector" -> [w314]
          tunnel: w122 -> [w313]
          tunnel: w121 -> [w312]
          n109 = case shown="\"T\"" w314 {
            tunnel: w321 -> [w329 w356 w369 w385 w395]
            tunnel: [w327 w344 w366 w383 w399] -> w319
            tunnel: [w333 w345 w367 w378 w400] -> w320
            tunnel: w318 -> [w327 _ _ _ _]
            tunnel: w317 -> [_ w344 _ _ _]
            tunnel: w316 -> [_ _ _ _ w399]
            tunnel: w315 -> [_ _ w366 _ _]
            tunnel: w313 -> [w322 w339 w363 w386 w396]
            tunnel: w312 -> [_ _ _ w383 _]
            frame "delay", Default {
              w335 = ":" ("string")
              n110 = local read "ESP_t0"() -> (w328:dbl)
              n111 = call "time2mm.vi"("fs[1]/ps[0]"=TRUE, "Offset (mm)"=w328, "time"=w329) -> ("position (mm)"=w324:dbl)
              n112 = local read "ESP Axis delay"() -> (w332:i32)
              n113 = Build Array(w324) -> (w323:dbl[])
              n114 = Number To Decimal String(number=w332) -> (decimal integer string=w331:string)  [unwired: 1 in]
              n115 = Number To Fractional String(number=w324) -> (F-format string=w337:string)  [unwired: 3 in]
              n116 = call-poly <vilib>:"Write Delimited Spreadsheet.vi"("file path (dialog if empty)"=w322, "format (%.3f)"="%.6f", "1D data"=w323, "append to file? (F)"=TRUE) -> ()  [unwired: 10 in, 2 out]
              n117 = Concatenate Strings("abs:" ("string"), w331, w335, w337, w335, "wait" ("string")) -> (w333:string)
            }
            frame "manip" {
              n118 = call-poly <vilib>:"Vector Norm.vi"("Input Vector"="scan_manip_deltas") -> ("norm"=w358:dbl)  [unwired: 9 in, 1 out]
              n119 = Divide(x="scan_manip_deltas", y=w358) -> (x/y=w357:dbl[])
              n120 = Multiply(x=w357, y=w356) -> (x*y=w342:dbl[])
              n121 = Add(x="scan_manip_start", y=w342) -> (x+y=w338:dbl[])
              n122 = call-poly <vilib>:"Write Delimited Spreadsheet.vi"("file path (dialog if empty)"=w339, "format (%.3f)"="%.6f", "1D data"=w338, "append to file? (F)"=TRUE) -> ()  [unwired: 10 in, 2 out]
              n123 = Index Array(array=w338) -> (element #1=w347:dbl, element #2=w348:dbl, element #3=w349:dbl, element #4=w350:dbl, element #5=w351:dbl, element #6=w352:dbl)  [unwired: 6 in]
              n124 = Format Into String(format string="%g_%g_%g_%g_%g_%g", w347, w348, w349, w350, w351, w352) -> (resulting string=w354:string)  [unwired: 2 in, 1 out]
              n125 = Concatenate Strings("abs:" ("string"), w354, ":wait" ("string")) -> (w345:string)
            }
            frame "mirror" {
              n126 = call-poly <vilib>:"Vector Norm.vi"("Input Vector"="scan_mirr_deltas") -> ("norm"=w377:dbl)  [unwired: 9 in, 1 out]
              n127 = Divide(x="scan_mirr_deltas", y=w377) -> (x/y=w376:dbl[])
              n128 = Multiply(x=w376, y=w369) -> (x*y=w365:dbl[])
              n129 = Add(x="scan_mirr_start", y=w365) -> (x+y=w362:dbl[])
              n130 = call-poly <vilib>:"Write Delimited Spreadsheet.vi"("file path (dialog if empty)"=w363, "format (%.3f)"="%.6f", "1D data"=w362, "append to file? (F)"=TRUE) -> ()  [unwired: 10 in, 2 out]
              n131 = Index Array(array=w362) -> (element #1=w372:dbl, element #2=w373:dbl)  [unwired: 2 in]
              n132 = Format Into String(format string="%g_%g", w372, w373) -> (resulting string=w375:string)  [unwired: 2 in, 1 out]
              n133 = Concatenate Strings("abs:" ("string"), w375, ":wait" ("string")) -> (w367:string)
            }
            frame "T" {
              n134 = Build Array(w385) -> (w384:dbl[])
              n135 = Number To Fractional String(number=w385) -> (F-format string=w382:string)  [unwired: 3 in]
              n136 = Concatenate Strings("ramp:" ("string"), w382) -> (w380:string)
              n137 = case shown="True" "Wait for T" {
                tunnel: w380 -> [w390 w393]
                tunnel: ":wait" ("string") -> [_ w392]
                tunnel: [w390 w391] -> w378
                frame False {
                }
                frame True {
                  n138 = Concatenate Strings(w393, w392) -> (w391:string)
                }
              }
              n139 = call-poly <vilib>:"Write Delimited Spreadsheet.vi"("file path (dialog if empty)"=w386, "format (%.3f)"="%.6f", "1D data"=w384, "append to file? (F)"=TRUE) -> ()  [unwired: 10 in, 2 out]
            }
            frame "volt" {
              n140 = local read "scan_volt_parameter"() -> (w403:string)
              n141 = Build Array(w395) -> (w394:dbl[])
              n142 = Number To Fractional String(number=w395) -> (F-format string=w401:string)  [unwired: 3 in]
              n143 = Concatenate Strings("setsgl:" ("string"), w403, ":" ("string"), w401) -> (w400:string)
              n144 = call-poly <vilib>:"Write Delimited Spreadsheet.vi"("file path (dialog if empty)"=w396, "format (%.3f)"="%.6f", "1D data"=w394, "append to file? (F)"=TRUE) -> ()  [unwired: 10 in, 2 out]
            }
          }
        }
        n145 = Build Path(base path=w139, name or relative path="RAW\\LUT.txt") -> (appended path=w137:path)
        n146 = call-poly <vilib>:"Write Delimited Spreadsheet.vi"("file path (dialog if empty)"=w137, "1D data"=string[] ["filename", "time", "delaystage", "X", "Y", "Z", "polar", "tilt", "azimuth", "mirrorX", "mirrorY", "KineticEnergy", "PassEnergy", "CoilCurrent", "WorkFunction", "DetectorVoltage", "ScreenVoltage", "ConversionVoltage", "FD1", "FD2"]) -> ("new file path (Not A Path if cancelled)"=w136:path)  [unwired: 12 in, 1 out]
        n147 = Get Date/Time In Seconds() -> (seconds since 1Jan1904=w149:timestamp)
        n148 = while {
          tunnel: w139 -> [w197]
          tunnel: w172 -> [w196]
          shift-right: [w195] -> w170
          shift-left: dbl[][][] [] -> [w194]
          tunnel: w169 -> [w193]
          tunnel: w149 -> [w192]
          tunnel: w142 -> [w191]
          tunnel: w141 -> [w190]
          tunnel: w140 -> [w189]
          shift-right: [w187] -> _
          shift-left: w136 -> [w188]
          shift-right: [w186] -> w134
          shift-left: w133 -> [w185]
          i -> [w184]
          stop <- w181 stop-if-true
          n149 = local read "meas_iter"() -> (w183:i32)
          n150 = for {
            N -> [w225]
            tunnel: w197 -> [w222]
            tunnel: w196 -> [w247]
            tunnel: w184 -> [w220]
            shift-right: [w236] -> w195
            shift-left: w194 -> [w243]
            tunnel: w193 -> [w238]
            tunnel: w192 -> [w224]
            tunnel: w191 -> [w216]
            tunnel: w190 -> [w215] mode=indexing
            tunnel: w189 -> [w214]
            shift-right: [w210] -> w187
            shift-left: w188 -> [w211]
            shift-right: [w206] -> w186
            shift-left: w185 -> [w206]
            tunnel: [w203] -> w180
            tunnel: w183 -> [w202]
            i -> [w221]
            stop <- "stop after step" stop-if-true
            n151 = Cancel Notification(0:w238) -> (11:w239:errorcluster)  [unwired: 1 in, 2 out]
            n152 = Enqueue Element(queue=w216, element=w215, error in (no error)=w239) -> (error out=w242:errorcluster)  [unwired: 1 in, 2 out]
            n153 = Equal To 0?(x=w221) -> (x = 0?=w246:bool)
            n154 = Equal To 0?(x=w220) -> (x = 0?=w245:bool)
            n155 = Get Date/Time In Seconds() -> (seconds since 1Jan1904=w212:timestamp)
            n156 = Wait on Notification(notifier=w238, error in (no error)=w242) -> (error out=w241:errorcluster)  [unwired: 2 in, 3 out]
            n157 = And(x=w246, y=w245) -> (x .and. y?=w244:bool)
            n158 = Enqueue Element(queue=w214, element="snap", error in (no error)=w241) -> (error out=w240:errorcluster)  [unwired: 1 in, 2 out]
            n159 = call "createFileStruc.vi"("i_iter"=w220, "i_delay"=w221, "meas_path"=w222) -> ("AVG file"=w217:path, "RAW file"=w208:path)  [unwired: 7 in]
            n160 = Dequeue Element(queue=w247, error in (no error)=w240) -> (element=w219:dbl[][], error out=w209:errorcluster)  [unwired: 1 in, 2 out]
            n161 = Strip Path(path=w208) -> (name=w207:string)  [unwired: 1 out]
            n162 = Array Size(array=w219) -> (size(s)=w251:i32[])
            n163 = call-poly <vilib>:"Write Delimited Spreadsheet.vi"("file path (dialog if empty)"=w208, "2D data"=w219, "error in (no error)"=w209) -> ()  [unwired: 11 in, 2 out]
            n164 = Index Array(array=w251) -> (element #1=w249:i32, element #2=w248:i32)  [unwired: 2 in]
            n165 = Subtract(x=w212, y=w224) -> (x-y=w228:dbl)
            n166 = flat-sequence {
              tunnel: "%s\\t%<%Y.%m.%d %H:%M:%S>T\\t%f\\t%f\\t%f\\t%f\\t%f\\t%f\\t%f\\t%f\\t%f\\t%f\\t%f\\t%f\\t%f\\t%f\\t%f\\t%f\\t%f\\t%f\\t%f" -> [w281]
              tunnel: w212 -> [w280]
              tunnel: w211 -> [w257]
              tunnel: [w256] -> w210
              tunnel: w209 -> [w253]
              tunnel: w207 -> [w252]
              frame #0 {
                n167 = local read "pos"() -> (w282:dbl[])
                n168 = local read "mirr_posX"() -> (w269:i32)
                n169 = local read "mirr_posY"() -> (w270:i32)
                n170 = local read "ESP_delay"() -> (w262:dbl)
                n171 = local read "phoib_I_1"() -> (w271:dbl)
                n172 = local read "phoib_I_2"() -> (w272:dbl)
                n173 = local read "phoib_I_3"() -> (w273:dbl)
                n174 = local read "phoib_I_4"() -> (w274:dbl)
                n175 = local read "phoib_I_5"() -> (w275:dbl)
                n176 = local read "phoib_I_6"() -> (w276:dbl)
                n177 = local read "phoib_I_7"() -> (w277:dbl)
                n178 = local read "phoib_I_8"() -> (w278:dbl)
                n179 = local read "phoib_I_9"() -> (w279:dbl)
                n180 = local read "ESP_pos"() -> (w261:dbl)
                n181 = Index Array(array=w282) -> (element #1=w263:dbl, element #2=w264:dbl, element #3=w265:dbl, element #4=w266:dbl, element #5=w267:dbl, element #6=w268:dbl)  [unwired: 6 in]
                n182 = Format Into String(format string=w281, error in=w253, w252, w280, w261, w262, w263, w264, w265, w266, w267, w268, w269, w270, w271, w272, w273, w274, w275, w276, w277, w278, w279) -> (resulting string=w259:string)  [unwired: 1 in, 1 out]
                n183 = Spreadsheet String To Array(format string="%s", spreadsheet string=w259, array type (2D Dbl)=string[] []) -> (array=w255:string[])  [unwired: 1 in]
                n184 = call-poly <vilib>:"Write Delimited Spreadsheet.vi"("file path (dialog if empty)"=w257, "1D data"=w255, "append to file? (F)"=TRUE) -> ("new file path (Not A Path if cancelled)"=w256:path)  [unwired: 11 in, 1 out]
              }
            }
            n185 = case shown="True" w244 {
              tunnel: w225 -> [_ w288]
              tunnel: [w283 w286] -> w250
              tunnel: w243 -> [w283 _]
              tunnel: w249 -> [_ w285]
              tunnel: w248 -> [_ w284]
              frame False {
              }
              frame True {
                n186 = Initialize Array(0.0 ("element"), w288, w285, w284) -> (w286:dbl[][][])
              }
            }
            n187 = Increment(x=w221) -> (x+1=w232:i32)
            "current scan" <- w232
            n188 = Increment(x=w220) -> (x+1=w231:i32)
            "current iteration" <- w231
            n189 = for {
              N: w249 -> [_]
              tunnel: w221 -> [w295]
              shift-right: [w293] -> w236
              shift-left: w250 -> [w296]
              tunnel: w220 -> [w291]
              shift-right: [w290] -> w218
              shift-left: w219 -> [w292]
              tunnel: w248 -> [w289]
              i -> [w294]
              n190 = for {
                N: w289 -> [_]
                tunnel: w295 -> [w303]
                tunnel: w294 -> [w300]
                shift-right: [w302] -> w293
                shift-left: w296 -> [w304]
                tunnel: w291 -> [w298]
                shift-right: [w297] -> w290
                shift-left: w292 -> [w301]
                i -> [w299]
                n191 = in-place {
                  in-place-border: w298 -> [w310]
                  n192 = in-place-array #1(w304, w303, w300, w299) -> (w311:dbl)
                  n193 = in-place-array #2(w301, w300, w299) -> (w308:dbl)
                  n194 = Multiply(x=w311, y=w310) -> (x*y=w309:dbl)
                  n195 = Increment(x=w310) -> (x+1=w306:i32)
                  n196 = Add(x=w309, y=w308) -> (x+y=w307:dbl)
                  n197 = Divide(x=w307, y=w306) -> (x/y=w305:dbl)
                  n198 = in-place-array #1(w305) -> (w302:dbl[][][])  [unwired: 3 out]
                  n199 = in-place-array #2(w305) -> (w297:dbl[][])  [unwired: 2 out]
                }
              }
            }
            n200 = Multiply(x=w225, y=w220) -> (x*y=w227:i32)
            n201 = Multiply(x=w225, y=w202) -> (x*y=w223:i32)
            n202 = Divide(x=w232, y=w225) -> (x/y=→"scan":dbl)
            n203 = Divide(x=w231, y=w202) -> (x/y=→"iteration":dbl)
            n204 = Add(x=w221, y=w227) -> (x+y=w226:i32)
            n205 = Divide(x=w228, y=w226) -> (x/y=w198:dbl)
            n206 = Multiply(x=w198, y=w223) -> (x*y=w201:dbl)
            n207 = local write "time/step [s]"(w198) -> ()
            n208 = local write "duration [HH:MM:SS]"(w201) -> ()
            n209 = property on="mainimg" class="IntGraph (strict)"() -> ("CrsrLis"=w235:T4)  [unwired: 2 in, 2 out]
            n210 = call-poly <vilib>:"Write Delimited Spreadsheet.vi"("file path (dialog if empty)"=w217, "2D data"=w218) -> ()  [unwired: 12 in, 2 out]
            n211 = call "processData.vi"("Cursor List"=w235, "data in"=w236) -> ("Angle Chart"=→"anglegraph":dbl[][], "Energy Chart"=→"energygraph":dbl[][], "Intensity Chart"=w234:dbl[])  [unwired: 1 in]
            n212 = Bundle("Array"=w206, "Intensity Chart"=w234) -> (→"intensitygraph":cluster{"Array":dbl[], "Intensity Chart":dbl[]})  [unwired: 1 in]
            n213 = Or(x="stop after iteration", y="stop after step") -> (x .or. y?=w203:bool)
          }
          n214 = Increment(x=w184) -> (x+1=w182:i32)
          n215 = Greater Or Equal?(x=w182, y=w183) -> (x >= y?=w179:bool)
          n216 = Or(x=w180, y=w179) -> (x .or. y?=w181:bool)
        }
      }
      frame "refresh" {
        n217 = Dequeue Element(queue=w410) -> ()  [unwired: 2 in, 4 out]
        n218 = property on="mainimg" class="IntGraph (strict)"() -> ("CrsrLis"=w417:T4)  [unwired: 2 in, 2 out]
        n219 = call "processData.vi"("Cursor List"=w417, "data in"=w416) -> ("Angle Chart"=w414:dbl[][], "Energy Chart"=w415:dbl[][], "Intensity Chart"=w411:dbl[])  [unwired: 1 in]
        n220 = Bundle("Array"=w412, "Intensity Chart"=w411) -> (w413:cluster{"Array":dbl[], "Intensity Chart":dbl[]})  [unwired: 1 in]
        n221 = local write "energygraph"(w415) -> ()
        n222 = local write "intensitygraph"(w413) -> ()
        n223 = local write "anglegraph"(w414) -> ()
      }
    }
  }
  n224 = while {
    tunnel: w20 -> [w426]
    tunnel: w19 -> [w425]
    tunnel: w18 -> [w424]
    tunnel: w17 -> [w423]
    tunnel: w22 -> [w421]
    tunnel: w29 -> [w422]
    tunnel: w5 -> [w420]
    tunnel: w10 -> [w419]
    tunnel: w1 -> [w418]
    stop <- w427 stop-if-true
    n225 = event shown="[1] \"main_close\": Value Change" {
      selector: _ -> [_ _ _ _ _ _ _ _ _ _ _ _ _ _ _ _ _ _ _ _ _ _ _ _ _ _ _ _ _ _ _]
      dyn-events: _ -> [_ _ _ _ _ _ _ _ _ _ _ _ _ _ _ _ _ _ _ _ _ _ _ _ _ _ _ _ _ _ _]
      timeout: _ -> [_ _ _ _ _ _ _ _ _ _ _ _ _ _ _ _ _ _ _ _ _ _ _ _ _ _ _ _ _ _ _]
      tunnel: [_ TRUE _ _ _ _ _ _ _ _ _ _ _ _ _ _ _ _ _ _ _ _ _ _ _ _ _ _ _ _ _] -> w427
      tunnel: w426 -> [_ w442 w454 _ _ _ _ _ _ w482 w484 _ _ _ _ _ _ _ _ _ _ _ _ _ _ _ _ _ _ _ _]
      tunnel: w425 -> [_ w441 _ w458 _ _ _ _ _ _ _ _ _ _ _ _ _ _ _ _ w550 _ _ w572 _ _ _ _ _ _ _]
      tunnel: w424 -> [_ w440 _ _ w464 _ _ _ _ _ _ _ _ _ _ _ _ w524 w540 w542 _ _ _ _ _ _ _ _ _ _ _]
      tunnel: w423 -> [_ w439 _ _ _ _ w472 w478 w479 _ _ _ _ _ _ _ _ _ _ _ _ _ _ _ _ _ _ _ _ _ _]
      tunnel: w422 -> [_ w447 _ _ _ _ _ _ _ _ _ _ _ _ _ _ _ _ _ _ _ _ _ _ _ _ _ _ _ _ _]
      tunnel: w421 -> [_ w438 _ _ _ _ _ _ _ _ _ w486 w488 _ _ _ _ _ _ _ _ _ _ _ _ _ _ _ w592 _ _]
      tunnel: w420 -> [_ w446 _ _ _ _ _ _ _ _ _ _ _ _ _ _ _ _ _ _ _ _ _ _ _ _ _ _ _ _ _]
      tunnel: w419 -> [_ w437 _ _ _ _ _ _ _ _ _ _ _ _ w502 _ _ _ _ _ _ _ _ _ _ _ _ _ _ w594 w615]
      tunnel: w418 -> [_ w430 _ _ _ _ _ _ _ _ _ _ _ _ _ _ _ _ _ _ _ _ _ _ _ _ _ _ _ _ _]
      event Timeout {
        n226 = event-data() -> ()  [unwired: 1 in, 1 out]
      }
      event "main_close": Value Change {
        w428 = "close" ("element")
        w443 = "release" ("element")
        n227 = event-data() -> ()  [unwired: 1 in, 1 out]
        n228 = Flush Queue(queue=w442) -> (queue out=w436:refnum<queue>)  [unwired: 1 in, 2 out]
        n229 = Flush Queue(queue=w441) -> (queue out=w435:refnum<queue>)  [unwired: 1 in, 2 out]
        n230 = Flush Queue(queue=w440) -> (queue out=w434:refnum<queue>)  [unwired: 1 in, 2 out]
        n231 = Flush Queue(queue=w439) -> (queue out=w433:refnum<queue>)  [unwired: 1 in, 2 out]
        n232 = Flush Queue(queue=w438) -> (queue out=w432:refnum<queue>)  [unwired: 1 in, 2 out]
        n233 = Flush Queue(queue=w437) -> (queue out=w431:refnum<queue>)  [unwired: 1 in, 2 out]
        n234 = Flush Queue(queue=w430) -> (queue out=w429:refnum<queue>)  [unwired: 1 in, 2 out]
        n235 = Release Notifier(notifier=w446) -> ()  [unwired: 2 in, 3 out]
        n236 = Release Queue(queue=w447) -> ()  [unwired: 2 in, 3 out]
        n237 = Enqueue Element(queue=w436, element=w443) -> (queue out=w451:refnum<queue>)  [unwired: 2 in, 2 out]
        n238 = Enqueue Element(queue=w435, element=w443) -> (queue out=w450:refnum<queue>)  [unwired: 2 in, 2 out]
        n239 = Enqueue Element(queue=w434, element=w443) -> (queue out=w449:refnum<queue>)  [unwired: 2 in, 2 out]
        n240 = Enqueue Element(queue=w433, element=w443) -> (queue out=w448:refnum<queue>)  [unwired: 2 in, 2 out]
        n241 = Enqueue Element(queue=w431, element=w443) -> (queue out=w445:refnum<queue>, error out=w444:errorcluster)  [unwired: 2 in, 1 out]
        n242 = Enqueue Element(queue=w451, element=w428) -> ()  [unwired: 2 in, 3 out]
        n243 = Enqueue Element(queue=w450, element=w428) -> ()  [unwired: 2 in, 3 out]
        n244 = Enqueue Element(queue=w449, element=w428) -> ()  [unwired: 2 in, 3 out]
        n245 = Enqueue Element(queue=w448, element=w428) -> ()  [unwired: 2 in, 3 out]
        n246 = Enqueue Element(queue=w432, element=w428) -> ()  [unwired: 2 in, 3 out]
        n247 = Enqueue Element(queue=w445, element=w428, error in (no error)=w444) -> ()  [unwired: 1 in, 3 out]
        n248 = Enqueue Element(queue=w429, element=w428) -> ()  [unwired: 2 in, 3 out]
      }
      event "cam_release", "cam_init": Value Change {
        n249 = event-data() -> ()  [unwired: 1 in, 2 out]
        n250 = Select(t="init" ("name (unnamed)"), s="cam_init", f="release" ("name (unnamed)")) -> (s? t:f=w453:string)
        n251 = Enqueue Element(queue=w454, element=w453) -> ()  [unwired: 2 in, 3 out]
      }
      event "ESP_release", "ESP_init": Value Change {
        n252 = event-data() -> ()  [unwired: 1 in, 2 out]
        n253 = Select(t="init" ("name (unnamed)"), s="ESP_init", f="release" ("name (unnamed)")) -> (s? t:f=w462:string)
        n254 = Enqueue Element(queue=w458, element=w462) -> ()  [unwired: 2 in, 3 out]
      }
      event "manip_init", "manip_release": Value Change {
        n255 = event-data() -> ()  [unwired: 1 in, 2 out]
        n256 = Flush Queue(queue=w464) -> (queue out=w463:refnum<queue>)  [unwired: 1 in, 2 out]
        n257 = Select(t="init" ("name (unnamed)"), s="manip_init", f="release" ("name (unnamed)")) -> (s? t:f=w466:string)
        n258 = Enqueue Element(queue=w463, element=w466) -> ()  [unwired: 2 in, 3 out]
      }
      event "setpoint_set": Value Change {
        n259 = event-data() -> ()  [unwired: 1 in, 2 out]
        n260 = local read "Setpoint"() -> (w470:dbl)
        n261 = local read "LS310  EPICS SP"() -> (w469:string)
        n262 = call-poly <userlib>:"CaLabPut.vi"("Value"=w470, "PV Name"=w469) -> ()  [unwired: 6 in, 4 out]
      }
      event "phoib_release", "phoib_init": Value Change {
        n263 = event-data() -> ()  [unwired: 1 in, 2 out]
        n264 = Flush Queue(queue=w472) -> (queue out=w471:refnum<queue>)  [unwired: 1 in, 2 out]
        n265 = Select(t="init" ("name (unnamed)"), s="phoib_init", f="release" ("name (unnamed)")) -> (s? t:f=w474:string)
        n266 = Enqueue Element(queue=w471, element=w474) -> ()  [unwired: 2 in, 3 out]
      }
      event "phoib_standby": Value Change {
        n267 = event-data() -> ()  [unwired: 1 in, 2 out]
        n268 = Enqueue Element(queue=w478, element="standby") -> ()  [unwired: 2 in, 3 out]
      }
      event "phoib_set": Value Change {
        n269 = event-data() -> ()  [unwired: 1 in, 2 out]
        n270 = Enqueue Element(queue=w479, element="set") -> ()  [unwired: 2 in, 3 out]
      }
      event "cam_dark": Value Change {
        n271 = event-data() -> ()  [unwired: 1 in, 2 out]
        n272 = Enqueue Element(queue=w482, element="dark") -> ()  [unwired: 2 in, 3 out]
      }
      event "ROI Left", "ROI Right", "ROI Top", "ROI Bottom", "cam_exp", "binning", "gain": Value Change {
        n273 = event-data() -> ()  [unwired: 1 in, 1 out]
        n274 = Enqueue Element(queue=w484, element="set") -> ()  [unwired: 2 in, 3 out]
      }
      event "cam_saveimg": Value Change {
        n275 = event-data() -> ()  [unwired: 1 in, 1 out]
        n276 = Enqueue Element(queue=w486, element="single") -> ()  [unwired: 2 in, 3 out]
      }
      event "scan_go": Value Change {
        n277 = event-data() -> ()  [unwired: 1 in, 1 out]
        n278 = Enqueue Element(queue=w488, element="scan") -> ()  [unwired: 2 in, 3 out]
      }
      event "meas_iter", "waypoints": Value Change {
        n279 = event-data() -> ()  [unwired: 1 in, 6 out]
        n280 = local read "waypoints"() -> (w500:string[][])
        n281 = local read "meas_iter"() -> (w494:i32)
        n282 = local read "binning"() -> (w497:u16)
        n283 = call "create scan vectr.vi"("Table Control"=w500) -> ("Array"=w499:dbl[])
        n284 = Index Array(array=dbl[] [8.79, 2.2, 0.553, 0.138], index=w497) -> (element=w493:dbl)
        n285 = Array Size(array=w499) -> (size(s)=w496:i32)
        "measpoints" <- w496
        n286 = Multiply(x=w496, y=w494) -> (x*y=w491:i32)
        "total steps" <- w491
        n287 = Multiply(x=w491, y="time/step [s]") -> (x*y=→"duration [HH:MM:SS]":dbl)
        n288 = Multiply(x=w496, y=w493) -> (x*y=→"RAM [MB]":dbl)
        n289 = Multiply(x=w491, y=w493) -> (x*y=→"disk [MB]":dbl)
      }
      event "mirr_go": Value Change {
        n290 = event-data() -> ()  [unwired: 1 in, 1 out]
        n291 = Index Array(array="mirr_dest") -> (element #1=w507:i32, element #2=w506:i32)  [unwired: 2 in]
        n292 = Format Into String(format string="%g_%g", w507, w506) -> (resulting string=w504:string)  [unwired: 2 in, 1 out]
        n293 = Concatenate Strings("abs:" ("string"), w504) -> (w501:string)
        n294 = Enqueue Element(queue=w502, element=w501) -> ()  [unwired: 2 in, 3 out]
      }
      event "scan_manip_setstart": Value Change {
        n295 = event-data() -> ()  [unwired: 1 in, 1 out]
        n296 = local read "pos"() -> (w509:dbl[])
        n297 = local write "scan_manip_start"(w509) -> ()
      }
      event "scan_mirr_setstart": Value Change {
        n298 = event-data() -> ()  [unwired: 1 in, 1 out]
        n299 = local read "mirr_posX"() -> (w512:i32)
        n300 = local read "mirr_posY"() -> (w511:i32)
        n301 = Build Array(w512, w511) -> (w510:i32[])
        n302 = local write "scan_mirr_start"(w510) -> ()
      }
      event "Move Abs": Value Change {
        n303 = event-data() -> ()  [unwired: 1 in, 1 out]
        n304 = Index Array(array="dest") -> (element #1=w522:dbl, element #2=w521:dbl, element #3=w520:dbl, element #4=w519:dbl, element #5=w518:dbl, element #6=w517:dbl)  [unwired: 6 in]
        n305 = Format Into String(format string="%g_%g_%g_%g_%g_%g", w522, w521, w520, w519, w518, w517) -> (resulting string=w515:string)  [unwired: 2 in, 1 out]
        n306 = Concatenate Strings("abs:" ("string"), w515) -> (w514:string)
        n307 = Enqueue Element(queue=w524, element=w514) -> ()  [unwired: 2 in, 3 out]
      }
      event "ManipRel +", "ManipRel -": Value Change {
        n308 = event-data() -> ()  [unwired: 1 in, 2 out]
        n309 = Negate(x="manip_deltas") -> (-x=w528:dbl[])
        n310 = Select(t="manip_deltas", s="ManipRel +", f=w528) -> (s? t:f=w526:dbl[])
        n311 = Index Array(array=w526) -> (element #1=w532:dbl, element #2=w533:dbl, element #3=w534:dbl, element #4=w535:dbl, element #5=w536:dbl, element #6=w537:dbl)  [unwired: 6 in]
        n312 = Format Into String(format string="%g_%g_%g_%g_%g_%g", w532, w533, w534, w535, w536, w537) -> (resulting string=w539:string)  [unwired: 2 in, 1 out]
        n313 = Concatenate Strings("rel:" ("string"), w539, ":wait" ("string")) -> (w530:string)
        n314 = Enqueue Element(queue=w540, element=w530) -> ()  [unwired: 2 in, 3 out]
      }
      event "stop manip": Value Change {
        n315 = event-data() -> ()  [unwired: 1 in, 1 out]
        n316 = Enqueue Element(queue=w542, element="stop") -> ()  [unwired: 2 in, 3 out]
      }
      event "ESP_go": Value Change {
        w544 = ":" ("string")
        n317 = event-data() -> ()  [unwired: 1 in, 1 out]
        n318 = local read "ESP Axis delay"() -> (w543:i32)
        n319 = Number To Decimal String(number=w543) -> (decimal integer string=w546:string)  [unwired: 1 in]
        n320 = Number To Fractional String(number="ESP_dest") -> (F-format string=w545:string)  [unwired: 3 in]
        n321 = Concatenate Strings("abs:" ("string"), w546, w544, w545, w544) -> (w549:string)
        n322 = Enqueue Element(queue=w550, element=w549) -> ()  [unwired: 2 in, 3 out]
      }
      event "ESP_set_t0": Value Change {
        n323 = event-data() -> ()  [unwired: 1 in, 1 out]
        n324 = Current VI's Path() -> (path=w561:path)
        n325 = Strip Path(path=w561) -> (stripped path=w559:path)  [unwired: 1 out]
        n326 = Strip Path(path=w559) -> (stripped path=w558:path)  [unwired: 1 out]
        n327 = local read "ESP_pos"() -> (w560:dbl)
        "ESP_t0" <- w560
        n328 = Number To Fractional String(number=w560) -> (F-format string=w553:string)  [unwired: 3 in]
        n329 = Build Path(base path=w558, name or relative path="t0.txt") -> (appended path=w555:path)
        n330 = Get Date/Time In Seconds() -> (seconds since 1Jan1904=w557:timestamp)
        n331 = Format Date/Time String(time format string (%c)="%Y.%m.%d %H:%M", seconds (now)=w557) -> (date/time string=w554:string)  [unwired: 1 in]
        n332 = Build Array(w554, w553) -> (w552:string[])
        n333 = call-poly <vilib>:"Write Delimited Spreadsheet.vi"("file path (dialog if empty)"=w555, "1D data"=w552, "append to file? (F)"=TRUE) -> ()  [unwired: 11 in, 2 out]
      }
      event "ESP_opent0file": Value Change {
        n334 = event-data() -> ()  [unwired: 1 in, 6 out]
        n335 = Current VI's Path() -> (path=w565:path)
        n336 = Strip Path(path=w565) -> (stripped path=w564:path)  [unwired: 1 out]
        n337 = Strip Path(path=w564) -> (stripped path=w566:path)  [unwired: 1 out]
        n338 = call <vilib>:"System Exec.vi"("wait until completion? (T)"=FALSE, "working directory"=w566, "command line"="notepad t0.txt") -> ()  [unwired: 5 in, 4 out]
      }
      event "ESP_+", "ESP_-": Value Change {
        n339 = event-data() -> ()  [unwired: 1 in, 6 out]
        n340 = local read "ESP Axis delay"() -> (w568:i32)
        n341 = Negate(x="ESP_delta") -> (-x=w575:dbl)
        n342 = Select(t="ESP_delta", s="ESP_+", f=w575) -> (s? t:f=w573:dbl)
        n343 = Number To Decimal String(number=w568) -> (decimal integer string=w571:string)  [unwired: 1 in]
        n344 = Number To Fractional String(number=w573) -> (F-format string=w569:string)  [unwired: 3 in]
        n345 = Concatenate Strings("rel:" ("string"), w571, ":" ("string"), w569) -> (w578:string)
        n346 = Enqueue Element(queue=w572, element=w578) -> ()  [unwired: 2 in, 3 out]
      }
      event "ESP_dest": Value Change {
        n347 = event-data() -> ()  [unwired: 1 in, 6 out]
        n348 = local read "ESP_dest"() -> (w582:dbl)
        n349 = local read "ESP_t0"() -> (w581:dbl)
        n350 = call "mm2time.vi"("fs?"=TRUE ("fs[1]/ps[0]"), "Offset (mm)"=w581, "distance (mm)"=w582) -> ("time in fs/ps seconds"=w579:dbl)
        n351 = local write "ESP_dest_t"(w579) -> ()
      }
      event "ESP_dest_t": Value Change {
        n352 = event-data() -> ()  [unwired: 1 in, 1 out]
        n353 = local read "ESP_t0"() -> (w585:dbl)
        n354 = call "time2mm.vi"("fs[1]/ps[0]"=TRUE, "Offset (mm)"=w585, "time"="ESP_dest_t") -> ("position (mm)"=w583:dbl)
        n355 = local write "ESP_dest"(w583) -> ()
      }
      event "load delay table": Value Change {
        n356 = event-data() -> ()  [unwired: 1 in, 6 out]
        n357 = call-poly <vilib>:"Read Delimited Spreadsheet.vi"() -> ("all rows"=w588:string[][], "error out"=w587:errorcluster)  [unwired: 10 in, 4 out]
        n358 = case shown="No Error" w587 {
          tunnel: w588 -> [w589 _]
          frame No Error {
            n359 = local write "waypoints"(w589) -> ()
          }
          frame Error {
          }
        }
      }
      event "clear delay table": Value Change {
        n360 = event-data() -> ()  [unwired: 1 in, 6 out]
        n361 = local write "waypoints"(string[][] []) -> ()
      }
      event "mainimg": Cursor Release {
        n362 = event-data() -> ()  [unwired: 1 in, 1 out]
        n363 = Enqueue Element(queue=w592, element="refresh") -> ()  [unwired: 2 in, 3 out]
      }
      event "mirr_init", "mirr_release": Value Change {
        n364 = event-data() -> ()  [unwired: 1 in, 6 out]
        n365 = Flush Queue(queue=w594) -> (queue out=w595:refnum<queue>)  [unwired: 1 in, 2 out]
        n366 = Select(t="init" ("name (unnamed)"), s="mirr_init", f="release" ("name (unnamed)")) -> (s? t:f=w596:string)
        n367 = Enqueue Element(queue=w595, element=w596) -> ()  [unwired: 2 in, 3 out]
      }
      event "mirr_X-", "mirr_X+", "mirr_Y+", "mirr_Y-": Value Change {
        n368 = event-data() -> ()  [unwired: 1 in, 1 out]
        n369 = local read "mirr_X#"() -> (w606:u8)
        n370 = local read "mirr_Y#"() -> (w605:u8)
        n371 = Or(x="mirr_X+", y="mirr_X-") -> (x .or. y?=w607:bool)
        n372 = Or(x="mirr_X-", y="mirr_Y-") -> (x .or. y?=w613:bool)
        n373 = Negate(x="mirr_rel") -> (-x=w612:i32)
        n374 = Select(t=w606, s=w607, f=w605) -> (s? t:f=w604:u8)
        n375 = Select(t=w612, s=w613, f="mirr_rel") -> (s? t:f=w601:i32)
        n376 = Number To Decimal String(number=w604) -> (decimal integer string=w603:string)  [unwired: 1 in]
        n377 = Number To Decimal String(number=w601) -> (decimal integer string=w600:string)  [unwired: 1 in]
        n378 = Concatenate Strings("rel:" ("string"), w603, ":" ("string"), w600) -> (w599:string)
        n379 = Enqueue Element(queue=w615, element=w599) -> ()  [unwired: 2 in, 3 out]
      }
    }
  }
  n380 = while {
    tunnel: w20 -> [w642]
    shift-right: [w636] -> _
    shift-left: _ -> [w635]
    shift-right: [w634] -> _
    shift-left: _ -> [w632]
    shift-right: [w633] -> _
    shift-left: _ -> [w631]
    shift-right: [w628] -> _
    shift-left: 0 -> [w629]
    shift-right: [w627] -> _
    shift-left: _ -> [w626]
    shift-right: [w625] -> _
    shift-left: _ -> [w624]
    tunnel: w29 -> [w623]
    shift-right: [w622] -> _
    shift-left: _ -> [w621]
    shift-right: [w619] -> _
    shift-left: _ -> [w618]
    shift-right: [w617] -> _
    shift-left: _ -> [w616]
    i -> [w620]
    stop <- w630 stop-if-true
    # "cam"
    n381 = Preview Queue Element(queue=w642, timeout in ms (-1)=w629) -> (queue out=w641:refnum<queue>, element=w640:string)  [unwired: 1 in, 2 out]
    n382 = Match Pattern(string=w640, regular expression=":") -> (before substring=w637:string, after substring=w638:string)  [unwired: 1 in, 2 out]
    n383 = case shown="\"suspend\"" w637 {
      tunnel: w641 -> [w654 w686 w719 w732 _ w820 w850 w915]
      tunnel: w638 -> [_ _ _ _ _ _ _ _]
      tunnel: [w648 w673 w718 w730 w773 w817 w835 w913] -> w636
      tunnel: w635 -> [_ _ w718 w730 w773 w817 w835 w913]
      tunnel: [w653 w687 u64 0 ("Hout") w729 w777 w818 w845 w912] -> w634
      tunnel: [w655 w688 w715 w728 w778 w819 w836 w911] -> w633
      tunnel: w632 -> [_ w690 w717 w729 w780 w822 w847 w912]
      tunnel: w631 -> [_ w689 _ w728 w779 w821 w846 w911]
      tunnel: [_ _ _ TRUE _ _ _ _] -> w630
      tunnel: [_ _ -1 _ _ _ _ -1] -> w628
      tunnel: [w647 w674 _ _ w787 _ _ _] -> w627
      tunnel: w626 -> [w647 w674 _ _ w786 _ _ _]
      tunnel: [w648 w676 w713 w727 w782 w811 w848 w910] -> w625
      tunnel: w624 -> [_ w676 w713 w727 w782 _ w848 w910]
      tunnel: w623 -> [_ _ _ _ _ _ w839 _]
      tunnel: [w645 w671 w712 w725 w740 w808 w842 w909] -> w622
      tunnel: w621 -> [w645 w671 w712 w725 w775 w808 w842 w909]
      tunnel: w620 -> [_ _ _ _ w748 _ _ _]
      tunnel: [w646 w672 w711 w726 w774 w807 w841 w908] -> w619
      tunnel: w618 -> [w646 w672 w711 w726 w747 w807 w841 w908]
      tunnel: [w644 w668 refnum<k21> refnum ("task out") w724 w733 w806 w832 w907] -> w617
      tunnel: w616 -> [_ w668 w710 w724 w733 w806 w833 w907]
      frame "init" {
        w648 = u16[][] []
        n384 = flat-sequence {
          tunnel: [w657] -> w652
          tunnel: [w658] -> w651
          tunnel: [w666] -> w653
          tunnel: [w667] -> w655
          tunnel: w652 -> [w667]
          tunnel: w651 -> [w666]
          frame #0 {
            n385 = local write "cam_con?"(FALSE ("cam_con?")) -> ()
          }
          frame #1 {
            n386 = call "SCInitBoard.vi"("boardnr"="board number") -> ("Hout"=w661:u32, "error out"=w662:errorcluster)  [unwired: 1 in, 1 out]
            n387 = call "SCSetupCamera.vi"("Handle"=w661, "error in (no error)"=w662) -> ("Hout"=w663:u64, "error out"=w664:errorcluster)  [unwired: 1 out]
            n388 = call "SCStopCOC.vi"("error in (no error)"=w664, "Stop mode"=0, "Handle"=w663) -> ("error out"=w657:errorcluster, "Hout"=w658:u64)
          }
          frame #2 {
            n389 = local write "cam_con?"(TRUE ("cam_con?")) -> ()
          }
        }
        n390 = Dequeue Element(queue=w654) -> (queue out=w650:refnum<queue>)  [unwired: 2 in, 3 out]
        n391 = Enqueue Element At Opposite End(queue=w650, element="set") -> ()  [unwired: 2 in, 3 out]
        n392 = call-poly <vilib>:"DAQmx Create Virtual Channel.vi"("lines"=tag "Dev3/port0/line0") -> ("task out"=w644:refnum<k21>)  [unwired: 13 in, 1 out]
      }
      frame "set" {
        n393 = Dequeue Element(queue=w686) -> ()  [unwired: 2 in, 4 out]
        n394 = call "SCStopCOC.vi"("error in (no error)"=w689, "Stop mode"=0, "Handle"=w690) -> ("error out"=w705:errorcluster, "Hout"=w704:u64)
        n395 = Bundle By Name(cluster=cluster{"Delay":dbl, "Exposure ":dbl} {"Delay"=0.0, "Exposure "=0.0} ("Delay and exposure"), "Exposure"="cam_exp") -> (w683:cluster{"Delay":dbl, "Exposure ":dbl})
        n396 = Bundle By Name(cluster=T5 {"Camera type"=0, "Operating mode\nHP & QE / HS & DiCam Pro "=0, "Frame trigger \n(High Performance and QE only)"=0, "Sequence trigger"=0, "Low Light\n(QE only)"=FALSE, "Gain"=FALSE, "Horzontal\nbinning"=0, "Vertical\nbinning "=0, "ROI Left"=1, "ROI Right"=20, "ROI Top"=1, "ROI Bottom"=15} ("Camera controls"), "Operating mode\nHP & QE / HS & DiCam Pro"="Operating mode\nHP & QE / HS & DiCam Pro", "Horzontal\nbinning"="binning", "Vertical\nbinning"="binning", "ROI Left"="ROI Left", "ROI Right"="ROI Right", "ROI Top"="ROI Top", "ROI Bottom"="ROI Bottom", "Gain"="gain", "Frame trigger \n(High Performance and QE only)"="Frame trigger \n(High Performance and QE only)") -> (w700:T5)
        n397 = call "New delay and exposure forma.vi"("Operating mode\nHP & QE / HS & DiCam Pro"="Operating mode\nHP & QE / HS & DiCam Pro", "Delay and exposure"=w683) -> ("Output table"=w701:string)  [unwired: 3 in]
        n398 = call "SCSetCoC.vi"("error in (no error)"=w705, "Delay and exposure table"=w701, "Camera controls"=w700, "Handle"=w704) -> ("error out"=w693:errorcluster, "Hout"=w692:u64)  [unwired: 1 out]
        n399 = call "SCGetImageSize.vi"("Handle"=w692, "error in (no error)"=w693) -> ("Hout"=w691:u64, "error out"=w675:errorcluster, "Horizontal size"=w680:i32, "Vertical size"=w679:i32)  [unwired: 2 out]
        n400 = Greater?(x=w680, y=w679) -> (0:w681:bool)
        n401 = Initialize Array(u16 0 ("dimension size"), w679, w680) -> (w673:u16[][])
        n402 = call "SCRun.vi"("error in (no error)"=w675, "Run mode"=0, "Handle"=w691) -> ("error out"=w688:errorcluster, "Hout"=w687:u64)  [unwired: 1 out]
        n403 = Select(t=w680, s=w681, f=w679) -> (s? t:f=w678:i32)
        n404 = property on="mainimg" class="IntGraph (strict)"("XScale.Maximum"=w678, "YScale.Maximum"=w678) -> ()  [unwired: 2 in, 2 out]
      }
      frame "release" {
        n405 = Dequeue Element(queue=w719) -> (queue out=w706:refnum<queue>)  [unwired: 2 in, 3 out]
        n406 = flat-sequence {
          tunnel: w717 -> [w721]
          tunnel: [w720] -> w714
          tunnel: [w723] -> w715
          tunnel: w714 -> [w723]
          frame #0 {
            n407 = call "SCCloseBoard.vi"("Handle"=w721) -> ("error out"=w720:errorcluster)  [unwired: 1 in, 2 out]
          }
          frame #1 {
            n408 = local write "cam_con?"(FALSE ("cam_con?")) -> ()
          }
        }
        n409 = Enqueue Element(queue=w706, element="suspend") -> ()  [unwired: 2 in, 3 out]
        n410 = call <vilib>:"DAQmx Clear Task.vi"("task in"=w710) -> ()  [unwired: 14 in, 1 out]
      }
      frame "close" {
        n411 = Release Queue(queue=w732) -> ()  [unwired: 2 in, 3 out]
      }
      frame "idle", Default {
        n412 = call "grabimg.vi"("array in"=w773, "error in"=w779, "Hin"=w780) -> ("error out"=w778:errorcluster, "imgdata"=w776:i32[][], "Hout"=w777:u64)  [unwired: 6 in]
        n413 = local read "lower threshold"() -> (w771:i32)
        n414 = case shown="False" "cam_dark?" {
          tunnel: w782 -> [_ w805]
          tunnel: [w802 w804] -> w772
          tunnel: w776 -> [w802 w803]
          frame False {
          }
          frame True {
            n415 = Subtract(x=w803, y=w805) -> (x-y=w804:dbl[][])
          }
        }
        n416 = call "filtr_b.vi"("threshold"=w771, "input array"=w772) -> ("output array"=w763:dbl[][])  [unwired: 9 in]
        n417 = call <vilib>:"High Resolution Relative Seconds.vi"() -> ("relative seconds"=w787:dbl)
        n418 = Subtract(x=w787, y=w786) -> (x-y=w785:dbl)
        n419 = Array Size(array=w763) -> (size(s)=w762:i32[])
        n420 = Reciprocal(x=w785) -> (1/x=→"cam_fps":dbl)
        n421 = Index Array(array=w762) -> (element #1=w757:i32, element #2=w756:i32)  [unwired: 2 in]
        n422 = Subtract(x=w748, y=w747) -> (x-y=w746:i32)
        n423 = Less Or Equal?(x="pics2avg", y=w746) -> (x <= y?=w769:bool)
        n424 = And(x="reset every n pics", y=w769) -> (x .and. y?=w767:bool)
        n425 = Not(x=w767) -> (.not. x?=w766:bool)
        n426 = call-poly <vilib>:"Ramp Pattern.vi"("start"=0.0, "end"=w757, "samples"=w757) -> ("Ramp Pattern"=w752:dbl[])  [unwired: 7 in, 1 out]
        n427 = call-poly <vilib>:"Ramp Pattern.vi"("start"=0.0, "end"=w756, "samples"=w756) -> ("Ramp Pattern"=w753:dbl[])  [unwired: 7 in, 1 out]
        n428 = property on="mainimg" class="IntGraph (strict)"() -> ("CrsrLis"=w745:T4)  [unwired: 2 in, 2 out]
        n429 = And(x="cam_liveavg", y=w766) -> (x .and. y?=w764:bool)
        n430 = case shown="False" w764 {
          tunnel: w763 -> [w792 w798]
          tunnel: [w792 w795] -> w740
          tunnel: w775 -> [_ w800]
          tunnel: w748 -> [w793 _]
          tunnel: [w793 w801] -> w774
          tunnel: w747 -> [_ w801]
          tunnel: w746 -> [_ w794]
          frame False {
          }
          frame True {
            n431 = Multiply(x=w800, y=w794) -> (x*y=w799:dbl[][])
            n432 = Increment(x=w794) -> (x+1=w796:i32)
            n433 = Add(x=w799, y=w798) -> (x+y=w797:dbl[][])
            n434 = Divide(x=w797, y=w796) -> (x/y=w795:dbl[][])
          }
        }
        "mainimg" <- w740
        n435 = Index Array(array=w745) -> (element #1=w743:T6, element #2=w744:T6)  [unwired: 2 in]
        n436 = Unbundle By Name(w743) -> ("Position.X"=w737:dbl, "Position.Y"=w739:dbl)
        n437 = Unbundle By Name(w744) -> ("Position.X"=w741:dbl, "Position.Y"=w742:dbl)
        n438 = Array Max & Min(array=w740) -> (max value=→"max":dbl)  [unwired: 3 out]
        n439 = Subtract(x=w742, y=w739) -> (x-y=w738:dbl)
        n440 = Subtract(x=w741, y=w737) -> (x-y=w736:dbl)
        n441 = Array Subset(array=w740, index (row)=w739, length (row)=w738) -> (w751:dbl[][])  [unwired: 2 in]
        n442 = Array Subset(array=w740, index (col)=w737, length (col)=w736) -> (w749:dbl[][])  [unwired: 2 in]
        n443 = Array Subset(array=w740, index (row)=w739, length (row)=w738, index (col)=w737, length (col)=w736) -> (w735:dbl[][])
        n444 = Transpose 2D Array(2D array=w751) -> (transposed array=w750:dbl[][])
        n445 = Add Array Elements(numeric array=w735) -> (sum=→"sum" →"Waveform Chart":dbl)
        n446 = for {
          tunnel: w749 -> [w789] mode=indexing
          tunnel: [w788] -> w759 mode=indexing
          n447 = Add Array Elements(numeric array=w789) -> (sum=w788:dbl)
        }
        n448 = for {
          tunnel: w750 -> [w791] mode=indexing
          tunnel: [w790] -> w758 mode=indexing
          n449 = Add Array Elements(numeric array=w791) -> (sum=w790:dbl)
        }
        n450 = Bundle("Ramp Pattern"=w753, w758) -> (→"G2 X":cluster{"Ramp Pattern":dbl[], dbl[]})  [unwired: 1 in]
        n451 = Bundle(w759, "Ramp Pattern"=w752) -> (→"G2 Y":cluster{dbl[], "Ramp Pattern":dbl[]})  [unwired: 1 in]
      }
      frame "dark" {
        n452 = Dequeue Element(queue=w820) -> ()  [unwired: 2 in, 4 out]
        n453 = Array Size(array=w817) -> (size(s)=w816:i32[])
        n454 = Index Array(array=w816) -> (element #1=w815:i32, element #2=w814:i32)  [unwired: 2 in]
        n455 = Initialize Array(0.0 ("element"), w815, w814) -> (w812:dbl[][])
        n456 = for {
          N: "dark avg" -> [_]
          tunnel: w822 -> [w830]
          tunnel: w821 -> [w829]
          tunnel: [w828] -> w819
          tunnel: w817 -> [w827]
          tunnel: [w826] -> w818
          shift-right: [w823] -> w810
          shift-left: w812 -> [w824]
          n457 = call "grabimg.vi"("array in"=w827, "error in"=w829, "Hin"=w830) -> ("error out"=w828:errorcluster, "imgdata"=w825:i32[][], "Hout"=w826:u64)  [unwired: 6 in]
          n458 = Add(x=w825, y=w824) -> (x+y=w823:dbl[][])
        }
        n459 = Divide(x=w810, y="dark avg") -> (x/y=w811:dbl[][])
      }
      frame "snap" {
        n460 = Dequeue Element(queue=w850) -> ()  [unwired: 2 in, 4 out]
        n461 = local read "cam_dark?"() -> (w849:bool)
        n462 = local read "cam_avgs"() -> (w844:i32)
        n463 = To Double Precision Float(number=w835) -> (double precision float=w834:dbl[][])
        n464 = Equal To 0?(x="aq.mode") -> (x = 0?=w837:bool)
        n465 = Get Date/Time In Seconds() -> (seconds since 1Jan1904=w840:timestamp)
        n466 = for {
          N: w844 -> [w862]
          shift-right: [w879] -> w845
          shift-left: w847 -> [w881]
          shift-right: [w867] -> w843
          shift-left: w846 -> [w880]
          tunnel: w849 -> [w877]
          tunnel: w848 -> [w876]
          tunnel: w835 -> [w875]
          tunnel: w840 -> [w871]
          tunnel: w837 -> [w855]
          shift-right: [w863] -> w831
          shift-left: w834 -> [w864]
          shift-right: [w853] -> w832
          shift-left: w833 -> [w853]
          i -> [w851]
          stop <- "abort acq." stop-if-true
          n467 = call "grabimg.vi"("array in"=w875, "error in"=w880, "Hin"=w881) -> ("error out"=w867:errorcluster, "imgdata"=w878:i32[][], "Hout"=w879:u64)  [unwired: 6 in]
          n468 = local read "lower threshold"() -> (w858:i32)
          n469 = Increment(x=w851) -> (x+1=w860:i32)
          "acq. imgs" <- w860
          n470 = Get Date/Time In Seconds() -> (seconds since 1Jan1904=w874:timestamp)
          n471 = case shown="True" w877 {
            tunnel: w878 -> [w903 w906]
            tunnel: w876 -> [_ w905]
            tunnel: [w903 w904] -> w857
            frame False {
            }
            frame True {
              n472 = Subtract(x=w906, y=w905) -> (x-y=w904:dbl[][])
            }
          }
          n473 = Divide(x=w860, y=w862) -> (x/y=→"snap_prog":dbl)
          n474 = Subtract(x=w874, y=w871) -> (x-y=w873:dbl)
          n475 = call "filtr_b.vi"("threshold"=w858, "input array"=w857) -> ("output array"=w856:dbl[][])  [unwired: 9 in]
          n476 = Divide(x=w873, y=w851) -> (x/y=w869:dbl)
          n477 = Multiply(x=w869, y=w862) -> (x*y=w872:dbl)
          n478 = Reciprocal(x=w869) -> (1/x=w868:dbl)
          n479 = case shown="True" "count?" {
            tunnel: w856 -> [w894 w896]
            tunnel: "e-size" -> [_ w898]
            tunnel: w858 -> [_ w897]
            tunnel: [w894 w895] -> w854
            frame False {
            }
            frame True {
              n480 = Array Size(array=w896) -> (size(s)=w900:i32[])
              n481 = call "findr.vi"("thresh"=w897, "esize"=w898, "inp array"=w896) -> ("locs"=w899:i32[][])  [unwired: 8 in]
              n482 = Index Array(array=w900) -> (element #1=w902:i32, element #2=w901:i32)  [unwired: 2 in]
              n483 = call "drawe.vi"("Ysize"=w902, "Xsize"=w901, "pos array"=w899) -> ("img out"=w895:i32[][])  [unwired: 8 in]
            }
          }
          n484 = Add(x=w872, y=w871) -> (x+y=→"ETA":timestamp)
          n485 = local write "cam_fps"(w868) -> ()
          n486 = local write "mainimg"(w856) -> ()
          n487 = case shown="True" w855 {
            tunnel: w854 -> [w884 w892]
            tunnel: w864 -> [w886 w891]
            tunnel: [w885 w889] -> w863
            tunnel: [w883 w888] -> w852
            tunnel: w851 -> [w882 w887]
            frame False {
              n488 = Add(x=w884, y=w886) -> (x+y=w885:dbl[][])
              n489 = Increment(x=w882) -> (x+1=w883:i32)
            }
            frame True {
              n490 = Multiply(x=w891, y=w887) -> (x*y=w893:dbl[][])
              n491 = Increment(x=w887) -> (x+1=w888:i32)
              n492 = Add(x=w892, y=w893) -> (x+y=w890:dbl[][])
              n493 = Divide(x=w890, y=w888) -> (x/y=w889:dbl[][])
            }
          }
          "Pics L" <- w852
          n494 = local write "sideimg"(w863) -> ()
        }
        n495 = Enqueue Element(queue=w839, element=w831, error in (no error)=w843) -> (error out=w836:errorcluster)  [unwired: 1 in, 2 out]
      }
      frame "suspend" {
        n496 = Dequeue Element(queue=w915) -> ()  [unwired: 2 in, 4 out]
      }
    }
    "cam_error" <- w633
  }
  n497 = while {
    tunnel: w10 -> [w924]
    shift-right: [w921] -> _
    shift-left: _ -> [w922]
    tunnel: w5 -> [w920]
    shift-right: [w919] -> _
    shift-left: _ -> [w918]
    shift-right: [w916] -> _
    shift-left: _ -> [w917]
    stop <- w923 stop-if-true
    # "mirr"
    n498 = Preview Queue Element(queue=w924, timeout in ms (-1)=w922) -> (queue out=w927:refnum<queue>, element=w928:string)  [unwired: 1 in, 2 out]
    n499 = Match Pattern(string=w928, regular expression=":") -> (before substring=w926:string, after substring=w925:string)  [unwired: 1 in, 2 out]
    n500 = case shown="\"abs\"" w926 {
      tunnel: w927 -> [w963 w973 w988 w992 w995 w1000 _]
      tunnel: w925 -> [w957 w974 _ _ _ _ _]
      tunnel: [_ _ _ TRUE _ _ _] -> w923
      tunnel: [_ _ _ _ -1 _ _] -> w921
      tunnel: w920 -> [w930 _ _ _ _ _ _]
      tunnel: [w949 w970 refnum<visa-resource-name> refnum ("VISA resource name out") w990 w994 w999 w1005] -> w919
      tunnel: w918 -> [w962 w972 w987 w990 w994 _ w1009]
      tunnel: [w934 w969 w986 w989 w993 w998 w1004] -> w916
      tunnel: w917 -> [w961 w971 _ w989 w993 _ w1008]
      frame "abs" {
        w945 = u8 20 items=["Echo"=55, "Home"=1, "Move Absolute"=20, "Move Relative"=21, "Move at Constant Speed"=22, "Renumber"=2, "Restore Settings"=36, "Stop"=23] ("Command")
        w960 = u8 20 items=["Echo"=55, "Home"=1, "Move Absolute"=20, "Move Relative"=21, "Move at Constant Speed"=22, "Renumber"=2, "Restore Settings"=36, "Stop"=23] ("Command")
        n501 = Dequeue Element(queue=w963) -> ()  [unwired: 2 in, 4 out]
        n502 = Match Pattern(string=w957, regular expression=":") -> (before substring=w947:string, after substring=w933:string)  [unwired: 1 in, 2 out]
        n503 = Equal?(x=w933, y="wait") -> (x = y?=w931:bool)
        n504 = Scan From String(format string="%g_%g", input string=w947) -> (output 1=w942:dbl, output 2=w941:dbl)  [unwired: 4 in, 3 out]
        n505 = local read "mirr_X#"() -> (w944:u8)
        n506 = Bundle("mirr_X#"=w944, "Command"=w960, w942, "Response Count"=1) -> (w956:T7)  [unwired: 1 in]
        n507 = local read "mirr_Y#"() -> (w943:u8)
        n508 = call "Request Command.vi"("error in (no error)"=w961, "Request"=w956, "VISA resource name"=w962) -> ("error out"=w938:errorcluster, "VISA resource name out"=w939:refnum<visa-resource-name>)  [unwired: 5 in, 2 out]
        n509 = Bundle("mirr_Y#"=w943, "Command"=w945, w941, "Response Count"=1) -> (w940:T8)  [unwired: 1 in]
        n510 = call "Request Command.vi"("error in (no error)"=w938, "Request"=w940, "VISA resource name"=w939) -> ("error out"=w936:errorcluster, "VISA resource name out"=w937:refnum<visa-resource-name>)  [unwired: 5 in, 2 out]
        n511 = local read "mirr_X#"() -> (w954:u8)
        n512 = call "zaber_readpos.vi"("error in (no error)"=w936, "axis"=w954, "VISA in"=w937) -> ("error out"=w950:errorcluster, "position"=w955:i32, "VISA out"=w951:refnum<visa-resource-name>)  [unwired: 6 in]
        n513 = local read "mirr_Y#"() -> (w952:u8)
        n514 = local write "mirr_posX"(w955) -> ()
        n515 = call "zaber_readpos.vi"("error in (no error)"=w950, "axis"=w952, "VISA in"=w951) -> ("error out"=w935:errorcluster, "position"=w953:i32, "VISA out"=w949:refnum<visa-resource-name>)  [unwired: 6 in]
        n516 = local write "mirr_posY"(w953) -> ()
        n517 = case shown="True" w931 {
          tunnel: w935 -> [w964 w968]
          tunnel: [w964 w967] -> w934
          tunnel: w930 -> [_ w966]
          frame False {
          }
          frame True {
            n518 = Send Notification(notification=TRUE, notifier=w966, error in (no error)=w968) -> (error out=w967:errorcluster)  [unwired: 1 out]
          }
        }
      }
      frame "rel" {
        w977 = u8 21 items=["Echo"=55, "Home"=1, "Move Absolute"=20, "Move Relative"=21, "Move at Constant Speed"=22, "Renumber"=2, "Restore Settings"=36, "Stop"=23] ("Command")
        n519 = Dequeue Element(queue=w973) -> ()  [unwired: 2 in, 4 out]
        n520 = Match Pattern(string=w974, regular expression=":") -> (before substring=w979:string, after substring=w978:string)  [unwired: 1 in, 2 out]
        n521 = Decimal String To Number(string=w979) -> (number=w981:i32)  [unwired: 2 in, 1 out]
        n522 = Decimal String To Number(string=w978) -> (number=w982:i32)  [unwired: 2 in, 1 out]
        n523 = Bundle(w981, "Command"=w977, w982, "Response Count"=1) -> (w975:T9)  [unwired: 1 in]
        n524 = call "Request Command.vi"("error in (no error)"=w971, "Request"=w975, "VISA resource name"=w972) -> ("error out"=w969:errorcluster, "VISA resource name out"=w970:refnum<visa-resource-name>)  [unwired: 5 in, 2 out]
      }
      frame "release" {
        n525 = Dequeue Element(queue=w988) -> (queue out=w984:refnum<queue>)  [unwired: 2 in, 3 out]
        n526 = Enqueue Element(queue=w984, element="suspend") -> ()  [unwired: 2 in, 3 out]
        n527 = call "Close.vi"("VISA resource name"=w987) -> ("error out"=w986:errorcluster)  [unwired: 9 in, 1 out]
      }
      frame "close" {
        n528 = Release Queue(queue=w992) -> ()  [unwired: 2 in, 3 out]
      }
      frame "suspend" {
        n529 = Dequeue Element(queue=w995) -> ()  [unwired: 2 in, 4 out]
      }
      frame "init" {
        n530 = Dequeue Element(queue=w1000) -> ()  [unwired: 2 in, 4 out]
        n531 = call "Initialize.vi"("VISA resource name"="mirr_VISA") -> ("error out"=w998:errorcluster, "VISA resource name out"=w999:refnum<visa-resource-name>)  [unwired: 8 in, 1 out]
      }
      frame "idle", Default {
        n532 = local read "mirr_X#"() -> (w1010:u8)
        n533 = call "zaber_readpos.vi"("error in (no error)"=w1008, "axis"=w1010, "VISA in"=w1009) -> ("error out"=w1006:errorcluster, "position"=→"mirr_posX":i32, "VISA out"=w1007:refnum<visa-resource-name>)  [unwired: 6 in]
        n534 = local read "mirr_Y#"() -> (w1003:u8)
        n535 = call "zaber_readpos.vi"("error in (no error)"=w1006, "axis"=w1003, "VISA in"=w1007) -> ("error out"=w1004:errorcluster, "position"=→"mirr_posY":i32, "VISA out"=w1005:refnum<visa-resource-name>)  [unwired: 6 in]
      }
    }
    "mirr_Error" <- w916
  }
  n536 = while {
    tunnel: w19 -> [w1019]
    shift-right: [w1017] -> _
    shift-left: _ -> [w1015]
    shift-right: [w1016] -> _
    shift-left: _ -> [w1014]
    shift-right: [w1012] -> _
    shift-left: 0 -> [w1013]
    tunnel: w5 -> [w1011]
    stop <- w1018 stop-if-true
    # "ESP"
    n537 = Preview Queue Element(queue=w1019, timeout in ms (-1)=w1013) -> (queue out=w1022:refnum<queue>, element=w1023:string)  [unwired: 1 in, 2 out]
    n538 = Match Pattern(string=w1023, regular expression=":") -> (before substring=w1021:string, after substring=w1020:string)  [unwired: 1 in, 2 out]
    n539 = case shown="\"suspend\"" w1021 {
      tunnel: w1022 -> [_ w1034 w1052 w1094 w1097 w1104 w1109]
      tunnel: w1020 -> [_ w1039 w1059 _ _ _ _]
      tunnel: [_ _ _ _ _ TRUE _] -> w1018
      tunnel: [w1026 w1041 w1053 w1092 refnum<visa-resource-name> refnum ("VISA resource name out") w1101 w1108] -> w1017
      tunnel: [w1025 w1042 w1051 w1091 w1099 w1102 w1107] -> w1016
      tunnel: w1015 -> [w1030 w1044 w1057 w1092 w1100 w1101 _]
      tunnel: w1014 -> [w1029 w1043 w1058 w1091 _ w1102 _]
      tunnel: [_ _ _ -1 _ _ _] -> w1012
      tunnel: w1011 -> [_ _ w1045 _ _ _ _]
      frame "idle", Default {
        n540 = local read "ESP Axis delay"() -> (w1027:i32)
        n541 = local read "ESP_t0"() -> (w1033:dbl)
        n542 = call "Read Actual Position.vi"("error in (no error)"=w1029, "Axis (1)"=w1027, "VISA resource name"=w1030) -> ("error out"=w1025:errorcluster, "Position (units)"=w1028:dbl, "VISA resource name out"=w1026:refnum<visa-resource-name>)  [unwired: 2 in]
        "ESP_pos" <- w1028
        n543 = call "mm2time.vi"("fs?"=TRUE, "Offset (mm)"=w1033, "distance (mm)"=w1028) -> ("time in fs/ps seconds"=→"ESP_delay":dbl)
      }
      frame "rel" {
        n544 = Match Pattern(string=w1039, regular expression=":") -> (before substring=w1038:string, after substring=w1037:string)  [unwired: 1 in, 2 out]
        n545 = Dequeue Element(queue=w1034) -> ()  [unwired: 2 in, 4 out]
        n546 = Decimal String To Number(string=w1038) -> (number=w1036:i32)  [unwired: 2 in, 1 out]
        n547 = Fract/Exp String To Number(string=w1037) -> (number=w1035:dbl)  [unwired: 3 in, 1 out]
        n548 = call "Move Relative.vi"("error in (no error)"=w1043, "Position (0 units)"=w1035, "Axis (1)"=w1036, "VISA resource name"=w1044) -> ("error out"=w1042:errorcluster, "VISA resource name out"=w1041:refnum<visa-resource-name>)  [unwired: 2 in]
      }
      frame "abs" {
        n549 = Dequeue Element(queue=w1052) -> ()  [unwired: 2 in, 4 out]
        n550 = Match Pattern(string=w1059, regular expression=":") -> (before substring=w1060:string, after substring=w1049:string)  [unwired: 1 in, 2 out]
        n551 = Match Pattern(string=w1049, regular expression=":") -> (before substring=w1048:string, after substring=w1047:string)  [unwired: 1 in, 2 out]
        n552 = Decimal String To Number(string=w1060) -> (number=w1056:i32)  [unwired: 2 in, 1 out]
        n553 = Fract/Exp String To Number(string=w1048) -> (number=w1046:dbl)  [unwired: 3 in, 1 out]
        n554 = call "Move Absolute.vi"("error in (no error)"=w1058, "Position (0 units)"=w1046, "Axis (1)"=w1056, "VISA resource name"=w1057) -> ("error out"=w1054:errorcluster, "VISA resource name out"=w1055:refnum<visa-resource-name>)  [unwired: 2 in]
        n555 = case shown="\"wait\"" w1047 {
          tunnel: w1056 -> [_ w1079]
          tunnel: w1055 -> [w1063 w1081]
          tunnel: w1054 -> [w1062 w1080]
          tunnel: [w1063 w1068] -> w1053
          tunnel: [w1062 w1076] -> w1051
          tunnel: w1045 -> [_ w1075]
          frame "", Default {
          }
          frame "wait" {
            n556 = while {
              tunnel: w1079 -> [w1090]
              shift-right: [w1087] -> w1078
              shift-left: w1081 -> [w1089]
              shift-right: [w1086] -> w1077
              shift-left: w1080 -> [w1088]
              stop <- w1085 stop-if-true
              n557 = call "Get Axis Motion Status.vi"("error in (no error)"=w1088, "Axis (1)"=w1090, "VISA resource name"=w1089) -> ("error out"=w1086:errorcluster, "Motion Done"=w1085:bool, "VISA resource name out"=w1087:refnum<visa-resource-name>)  [unwired: 2 in]
            }
            n558 = flat-sequence {
              tunnel: w1078 -> [w1084]
              tunnel: w1077 -> [w1083]
              tunnel: [w1084] -> w1070
              tunnel: [w1083] -> w1069
              frame #0 {
                n559 = Wait (ms)(milliseconds to wait=u32 1000) -> ()  [unwired: 1 out]
              }
            }
            n560 = local read "ESP Axis delay"() -> (w1071:i32)
            n561 = local read "ESP_t0"() -> (w1073:dbl)
            n562 = call "Read Actual Position.vi"("error in (no error)"=w1069, "Axis (1)"=w1071, "VISA resource name"=w1070) -> ("error out"=w1064:errorcluster, "Position (units)"=w1066:dbl, "VISA resource name out"=w1068:refnum<visa-resource-name>)  [unwired: 2 in]
            n563 = call "mm2time.vi"("fs?"=TRUE, "Offset (mm)"=w1073, "distance (mm)"=w1066) -> ("time in fs/ps seconds"=w1067:dbl)
            n564 = call <vilib>:"Clear Errors.vi"("error in (no error)"=w1064) -> ("error out"=w1065:errorcluster)  [unwired: 5 in, 1 out]
            n565 = local write "ESP_pos"(w1066) -> ()
            n566 = local write "ESP_delay"(w1067) -> ()
            n567 = Send Notification(notification=TRUE, notifier=w1075, error in (no error)=w1065) -> (error out=w1076:errorcluster)  [unwired: 1 out]
          }
        }
      }
      frame "suspend" {
        n568 = Dequeue Element(queue=w1094) -> ()  [unwired: 2 in, 4 out]
      }
      frame "release" {
        n569 = Dequeue Element(queue=w1097) -> (queue out=w1095:refnum<queue>)  [unwired: 2 in, 3 out]
        n570 = call "Close.vi"("VISA resource name"=w1100) -> ("error out"=w1099:errorcluster)  [unwired: 10 in]
        n571 = Enqueue Element(queue=w1095, element="suspend") -> ()  [unwired: 2 in, 3 out]
      }
      frame "close" {
        n572 = Release Queue(queue=w1104) -> ()  [unwired: 2 in, 3 out]
      }
      frame "init" {
        n573 = Dequeue Element(queue=w1109) -> ()  [unwired: 2 in, 4 out]
        n574 = flat-sequence {
          tunnel: [w1112] -> w1106
          tunnel: [w1111] -> w1105
          tunnel: [w1116] -> w1107
          tunnel: [w1117] -> w1108
          tunnel: w1106 -> [w1117]
          tunnel: w1105 -> [w1116]
          frame #0 {
            n575 = local write "ESP_con?"(FALSE ("ESP_con?")) -> ()
          }
          frame #1 {
            n576 = call "Initialize.vi"("VISA resource name"="ESP301 VISA", "Serial Link (RS232)"=enum16{"RS232", "USB"}."RS232") -> ("VISA resource name out"=w1112:refnum<visa-resource-name>, "error out"=w1111:errorcluster)  [unwired: 7 in]
          }
          frame #2 {
            n577 = local write "ESP_con?"(TRUE ("ESP_con?")) -> ()
          }
        }
      }
    }
    "error out" <- w1016
  }
  n578 = while {
    tunnel: w18 -> [w1126]
    shift-right: [w1124] -> _
    shift-left: _ -> [w1122]
    shift-right: [w1123] -> _
    shift-left: _ -> [w1121]
    shift-right: [w1119] -> _
    shift-left: 0 -> [w1120]
    tunnel: w5 -> [w1118]
    stop <- w1125 stop-if-true
    # "manip"
    n579 = Preview Queue Element(queue=w1126, timeout in ms (-1)=w1120) -> (queue out=w1129:refnum<queue>, element=w1130:string)  [unwired: 1 in, 2 out]
    n580 = Match Pattern(string=w1130, regular expression=":") -> (before substring=w1128:string, after substring=w1127:string)  [unwired: 1 in, 2 out]
    n581 = case shown="\"init\"" w1128 {
      tunnel: w1129 -> [_ w1142 w1169 w1216 w1254 w1260 w1269 w1274]
      tunnel: w1127 -> [_ _ w1156 w1215 _ _ _ _]
      tunnel: [_ _ _ _ _ _ TRUE _] -> w1125
      tunnel: [w1136 w1144 w1148 w1213 w1256 refnum<k5> refnum ("gateway_connection out") w1267 w1273] -> w1124
      tunnel: [w1135 w1143 w1150 w1212 w1255 w1262 w1266 w1272] -> w1123
      tunnel: w1122 -> [w1138 w1146 w1172 w1206 w1256 w1264 w1267 _]
      tunnel: w1121 -> [w1137 w1145 w1171 w1207 w1255 _ w1266 _]
      tunnel: [_ _ _ _ -1 _ _ _] -> w1119
      tunnel: w1118 -> [_ _ w1147 w1209 _ _ _ _]
      frame "idle", Default {
        n582 = call "sp_manip_get_axis_status.vi"("error in"=w1137, "gateway_connection"=w1138) -> ("error out"=w1135:errorcluster, "axis_out"=w1134:T10, "gateway_connection out"=w1136:refnum<k5>)  [unwired: 5 in, 2 out]
        n583 = for {
          tunnel: w1134 -> [w1141] mode=indexing
          tunnel: [w1140] -> w1133 mode=indexing
          tunnel: [w1139] -> w1132 mode=indexing
          n584 = Unbundle By Name(w1141) -> ("Axis_Position"=w1140:dbl, "moving"=w1139:bool)
        }
        "moving?" <- w1132
        n585 = local write "pos"(w1133) -> ()
      }
      frame "stop" {
        n586 = Dequeue Element(queue=w1142) -> ()  [unwired: 2 in, 4 out]
        n587 = call "sp_manip_abort.vi"("error in"=w1145, "gateway_connection"=w1146) -> ("error out"=w1143:errorcluster, "gateway_connection out"=w1144:refnum<k5>)  [unwired: 6 in, 2 out]
      }
      frame "rel" {
        n588 = Dequeue Element(queue=w1169) -> ()  [unwired: 2 in, 4 out]
        n589 = Match Pattern(string=w1156, regular expression=":") -> (before substring=w1155:string, after substring=w1154:string)  [unwired: 1 in, 2 out]
        n590 = Equal?(x=w1154, y="wait") -> (x = y?=w1152:bool)
        n591 = call "sp_manip_get_axis_status.vi"("error in"=w1171, "gateway_connection"=w1172) -> ("error out"=w1174:errorcluster, "axis_out"=w1161:T10, "gateway_connection out"=w1173:refnum<k5>)  [unwired: 5 in, 2 out]
        n592 = Scan From String(format string="%g_%g_%g_%g_%g_%g", input string=w1155) -> (output 1=w1168:dbl, output 2=w1167:dbl, output 3=w1166:dbl, output 4=w1165:dbl, output 5=w1164:dbl, output 6=w1163:dbl)  [unwired: 8 in, 3 out]
        n593 = for {
          tunnel: w1161 -> [w1201] mode=indexing
          tunnel: [w1200] -> w1159 mode=indexing
          tunnel: [w1199] -> w1160 mode=indexing
          n594 = Unbundle By Name(w1201) -> ("Axis_Name"=w1200:string, "Axis_Position"=w1199:dbl)
        }
        n595 = Build Array(w1168, w1167, w1166, w1165, w1164, w1163) -> (w1162:dbl[])
        n596 = Add(x=w1160, y=w1162) -> (x+y=w1158:dbl[])
        n597 = call "sp_manip_start_move.vi"("error in"=w1174, "target positions"=w1158, "axis names"=w1159, "gateway_connection"=w1173) -> ("error out"=w1151:errorcluster, "gateway_connection out"=w1149:refnum<k5>)  [unwired: 4 in, 2 out]
        n598 = case shown="True" w1152 {
          tunnel: w1151 -> [w1175 w1186]
          tunnel: [w1175 w1185] -> w1150
          tunnel: w1149 -> [w1176 w1187]
          tunnel: [w1176 w1179] -> w1148
          tunnel: w1147 -> [_ w1184]
          frame False {
          }
          frame True {
            n599 = while {
              tunnel: w1187 -> [w1193]
              tunnel: w1186 -> [w1192]
              tunnel: [w1191] -> w1180
              tunnel: [w1190] -> w1178
              stop <- w1194 continue-if-true
              n600 = call "sp_manip_get_axis_status.vi"("error in"=w1192, "gateway_connection"=w1193) -> ("error out"=w1190:errorcluster, "axis_out"=w1196:T10, "gateway_connection out"=w1191:refnum<k5>)  [unwired: 5 in, 2 out]
              n601 = for {
                tunnel: w1196 -> [w1198] mode=indexing
                tunnel: [w1197] -> w1195 mode=indexing
                n602 = Unbundle By Name(w1198) -> ("moving"=w1197:bool)
              }
              n603 = Or Array Elements(Boolean array=w1195) -> (logical OR=w1194:bool)
            }
            n604 = call "sp_manip_get_axis_status.vi"("error in"=w1178, "gateway_connection"=w1180) -> ("error out"=w1177:errorcluster, "axis_out"=w1182:T10, "gateway_connection out"=w1179:refnum<k5>)  [unwired: 5 in, 2 out]
            n605 = for {
              tunnel: w1182 -> [w1189] mode=indexing
              tunnel: [w1188] -> w1181 mode=indexing
              n606 = Unbundle By Name(w1189) -> ("Axis_Position"=w1188:dbl)
            }
            n607 = Send Notification(notification=TRUE, notifier=w1184, error in (no error)=w1177) -> (error out=w1185:errorcluster)  [unwired: 1 out]
            n608 = local write "dest"(w1181) -> ()
          }
        }
      }
      frame "abs" {
        n609 = Dequeue Element(queue=w1216) -> ()  [unwired: 2 in, 4 out]
        n610 = call "sp_manip_get_axis_status.vi"("error in"=w1207, "gateway_connection"=w1206) -> ("error out"=w1202:errorcluster, "axis_out"=w1205:T10, "gateway_connection out"=w1203:refnum<k5>)  [unwired: 5 in, 2 out]
        n611 = Match Pattern(string=w1215, regular expression=":") -> (before substring=w1219:string, after substring=w1218:string)  [unwired: 1 in, 2 out]
        n612 = Equal?(x=w1218, y="wait") -> (x = y?=w1208:bool)
        n613 = for {
          tunnel: w1205 -> [w1229] mode=indexing
          tunnel: [w1228] -> w1204 mode=indexing
          n614 = Unbundle By Name(w1229) -> ("Axis_Name"=w1228:string)
        }
        n615 = Scan From String(format string="%g_%g_%g_%g_%g_%g", input string=w1219) -> (output 1=w1225:dbl, output 2=w1224:dbl, output 3=w1223:dbl, output 4=w1222:dbl, output 5=w1221:dbl, output 6=w1220:dbl)  [unwired: 8 in, 3 out]
        n616 = Build Array(w1225, w1224, w1223, w1222, w1221, w1220) -> (w1227:dbl[])
        n617 = call "sp_manip_start_move.vi"("error in"=w1202, "target positions"=w1227, "axis names"=w1204, "gateway_connection"=w1203) -> ("error out"=w1211:errorcluster, "gateway_connection out"=w1210:refnum<k5>)  [unwired: 4 in, 2 out]
        n618 = case shown="True" w1208 {
          tunnel: w1211 -> [w1230 w1241]
          tunnel: [w1230 w1240] -> w1212
          tunnel: w1210 -> [w1231 w1242]
          tunnel: [w1231 w1233] -> w1213
          tunnel: w1209 -> [_ w1239]
          frame False {
          }
          frame True {
            n619 = while {
              tunnel: w1242 -> [w1248]
              tunnel: w1241 -> [w1247]
              tunnel: [w1246] -> w1235
              tunnel: [w1245] -> w1234
              stop <- w1249 continue-if-true
              n620 = call "sp_manip_get_axis_status.vi"("error in"=w1247, "gateway_connection"=w1248) -> ("error out"=w1245:errorcluster, "axis_out"=w1251:T10, "gateway_connection out"=w1246:refnum<k5>)  [unwired: 5 in, 2 out]
              n621 = for {
                tunnel: w1251 -> [w1253] mode=indexing
                tunnel: [w1252] -> w1250 mode=indexing
                n622 = Unbundle By Name(w1253) -> ("moving"=w1252:bool)
              }
              n623 = Or Array Elements(Boolean array=w1250) -> (logical OR=w1249:bool)
            }
            n624 = call "sp_manip_get_axis_status.vi"("error in"=w1234, "gateway_connection"=w1235) -> ("error out"=w1232:errorcluster, "axis_out"=w1237:T10, "gateway_connection out"=w1233:refnum<k5>)  [unwired: 5 in, 2 out]
            n625 = for {
              tunnel: w1237 -> [w1244] mode=indexing
              tunnel: [w1243] -> w1236 mode=indexing
              n626 = Unbundle By Name(w1244) -> ("Axis_Position"=w1243:dbl)
            }
            n627 = local write "pos"(w1236) -> ()
            n628 = Send Notification(notification=TRUE, notifier=w1239, error in (no error)=w1232) -> (error out=w1240:errorcluster)  [unwired: 1 out]
          }
        }
      }
      frame "suspend" {
        n629 = Dequeue Element(queue=w1254) -> ()  [unwired: 2 in, 4 out]
      }
      frame "release" {
        n630 = Dequeue Element(queue=w1260) -> (queue out=w1258:refnum<queue>)  [unwired: 2 in, 3 out]
        n631 = call "sp_manip_disconnect.vi"("gateway_connection"=w1264) -> ("error out"=w1263:errorcluster, "gateway_connection_out"=w1265:refnum<k5>)  [unwired: 7 in, 2 out]
        n632 = call "tcp_gateway_close_connection.vi"("error in"=w1263, "server_connection"=w1265) -> ("error out"=w1262:errorcluster)  [unwired: 5 in]
        n633 = Enqueue Element(queue=w1258, element="suspend") -> ()  [unwired: 2 in, 3 out]
      }
      frame "close" {
        n634 = Release Queue(queue=w1269) -> ()  [unwired: 2 in, 3 out]
      }
      frame "init" {
        n635 = Dequeue Element(queue=w1274) -> ()  [unwired: 2 in, 4 out]
        n636 = flat-sequence {
          tunnel: [w1277] -> w1271
          tunnel: [w1276] -> w1270
          tunnel: [w1287] -> w1272
          tunnel: [w1288] -> w1273
          tunnel: w1271 -> [w1288]
          tunnel: w1270 -> [w1287]
          frame #0 {
            n637 = local write "manip_con?"(FALSE ("manip_con?")) -> ()
          }
          frame #1 {
            n638 = call "tcp_gateway_open_connection.vi"() -> ("gateway_connection"=w1280:refnum<k5>, "error out"=w1279:errorcluster)  [unwired: 5 in, 3 out]
            n639 = call "sp_manip_connect.vi"("error in"=w1279, "gateway_connection"=w1280) -> ("error out"=w1276:errorcluster, "axis_out"=w1278:T10, "gateway_connection out"=w1277:refnum<k5>)  [unwired: 5 in, 2 out]
            n640 = for {
              tunnel: w1278 -> [w1285] mode=indexing
              tunnel: [w1284] -> w1281 mode=indexing
              tunnel: [w1283] -> w1282 mode=indexing
              n641 = Unbundle By Name(w1285) -> ("Axis_Name"=w1284:string, "Axis_Position"=w1283:dbl)
            }
            "axis" <- w1281
            "pos" <- w1282
            n642 = local write "dest"(w1282) -> ()
          }
          frame #2 {
            n643 = local write "manip_con?"(TRUE ("manip_con?")) -> ()
          }
        }
      }
    }
    "error out 2" <- w1123
  }
  n644 = while {
    tunnel: w17 -> [w1300]
    shift-right: [w1289] -> _
    shift-left: 0 -> [w1298]
    shift-right: [w1297] -> _
    shift-left: _ -> [w1296]
    shift-right: [w1295] -> _
    shift-left: _ -> [w1294]
    shift-right: [w1293] -> _
    shift-left: u32 0 ("pHandle") -> [w1292]
    tunnel: w15 -> [w1291]
    tunnel: w5 -> [w1290]
    stop <- w1299 stop-if-true
    # "phoib"
    n645 = Preview Queue Element(queue=w1300, timeout in ms (-1)=w1298) -> (queue out=w1303:refnum<queue>, element=w1304:string)  [unwired: 1 in, 2 out]
    n646 = Match Pattern(string=w1304, regular expression=":") -> (before substring=w1302:string, after substring=w1301:string)  [unwired: 1 in, 2 out]
    n647 = case shown="\"init\"" w1302 {
      tunnel: w1303 -> [_ w1361 w1416 w1433 w1451 w1465 w1470 w1475]
      tunnel: w1301 -> [_ _ w1412 _ _ _ _ _]
      tunnel: [_ _ _ _ _ TRUE _ _] -> w1299
      tunnel: [w1315 w1363 w1381 w1436 w1449 w1463 w1469 w1472] -> w1297
      tunnel: w1296 -> [w1326 w1352 w1402 w1438 w1450 w1463 w1469 _]
      tunnel: [w1314 w1362 w1397 w1435 w1448 w1461 w1467 w1471] -> w1295
      tunnel: w1294 -> [w1324 w1351 _ w1437 _ w1461 w1467 _]
      tunnel: [w1312 w1349 w1380 w1434 w1447 w1462 w1468 w1474] -> w1293
      tunnel: w1292 -> [w1312 w1349 w1400 w1434 w1446 w1462 w1468 _]
      tunnel: w1291 -> [w1313 w1342 w1378 _ _ _ _ _]
      tunnel: w1290 -> [_ _ w1396 _ _ _ _ _]
      tunnel: [_ _ _ _ _ _ -1 _] -> w1289
      frame "idle", Default {
        n648 = call "SL2_AD_DLL_Phoibos_GetDeviceState.vi"("dll_path"=w1326, "pHandle_in"=w1312, "dev_type"=DEF_dev_type."devA (analyzer)", "error in"=w1324) -> ("path out"=w1311:path, "state"=→"state":T2, "error out"=w1310:errorcluster)  [unwired: 2 in]
        n649 = for {
          tunnel: w1312 -> [w1333]
          tunnel: w1313 -> [w1331] mode=indexing
          tunnel: [w1330] -> w1323 mode=indexing
          tunnel: [w1329] -> w1315
          shift-right: [w1328] -> w1314
          shift-left: w1310 -> [w1332]
          tunnel: w1311 -> [w1327]
          n650 = call "SL2_AD_DLL_Phoibos_GetVoltage.vi"("error in"=w1332, "voltage_name"=w1331, "pHandle"=w1333, "dll path in"=w1327) -> ("error out"=w1328:errorcluster, "value"=w1330:dbl, "dll path out"=w1329:path)  [unwired: 3 in]
        }
        n651 = Index Array(array=w1323) -> (element #1=→"phoib_I_1":dbl, element #2=→"phoib_I_2":dbl, element #3=→"phoib_I_3":dbl, element #4=→"phoib_I_4":dbl, element #5=→"phoib_I_5":dbl, element #6=→"phoib_I_6":dbl, element #7=→"phoib_I_7":dbl, element #8=→"phoib_I_8":dbl, element #9=→"phoib_I_9":dbl, element #10=→"phoib_I_10":dbl)  [unwired: 10 in]
      }
      frame "set" {
        n652 = Dequeue Element(queue=w1361) -> ()  [unwired: 2 in, 4 out]
        n653 = Add(x=u32[] [251749632, 251749633, 251749634, 251749635, 251749636, 251749637, 251749638, 251749639, 251749640, 251749641, 251749642, 251749643, 251749644, 251749645, 251749646, 251749647, 251749648, 251749649, 251749650, 251749651, 251749652, 251749653, 251749654, 251749655, 251749656, 251749657, 251749658, 251749659, 251749660, 251749661, 251749662, 251749663, 251749664, 251749665, 251749666, 251749667, 251749668, 251749669, 251749670, 251749671, 251749672, 251749673, 251749674, 251749675, 251749676, 251749677, 251749678, 251749679, 251749680, 251749681, 251749682, 251749683, 251749684, 251749685, 251749686, 251749687, 251749688, 251749689, 251749690, 251749691, 251749692, 251749693, 251749694, 251749695, 251749696] ("modeIDs"), y=9984) -> (x+y=w1335:u32[])
        n654 = Multiply(x="ana_voltrange", y=12) -> (x*y=w1358:i32)
        n655 = Add(x="ana_mode", y=w1358) -> (x+y=w1355:i32)
        n656 = Index Array(array=w1335, index=w1355) -> (element=w1353:u32)
        n657 = Build Array("phoib_I_1s", "phoib_I_2s", "phoib_I_3s", "phoib_I_4s", "phoib_I_5s", "phoib_I_6s", "phoib_I_7s", "phoib_I_8s", "phoib_I_9s", "phoib_I_10s") -> (w1341:dbl[])
        n658 = call "SL2_AD_DLL_Phoibos_SetDeviceMode.vi"("pHandle"=w1349, "error in"=w1351, "value"=w1353, "dev_type"=DEF_dev_type."devA (analyzer)", "dll path in"=w1352) -> ("error out"=w1340:errorcluster, "dll path out"=w1350:path)  [unwired: 4 in]
        n659 = for {
          tunnel: w1349 -> [w1369]
          shift-right: [w1376] -> w1363
          shift-left: w1350 -> [w1373]
          tunnel: w1342 -> [w1368] mode=indexing
          tunnel: w1341 -> [w1367] mode=indexing
          shift-right: [w1375] -> w1362
          shift-left: w1340 -> [w1371]
          n660 = call "SL2_AD_DLL_Phoibos_GetVoltageRange.vi"("error in"=w1371, "voltage_name"=w1368, "pHandle"=w1369, "dll path in"=w1373) -> ("error out"=w1370:errorcluster, "min"=w1365:dbl, "max"=w1366:dbl, "dll path out"=w1372:path)  [unwired: 2 in]
          n661 = In Range and Coerce(upper limit=w1366, x=w1367, lower limit=w1365) -> (coerced(x)=w1364:dbl)  [unwired: 1 out]
          n662 = call "SL2_AD_DLL_Phoibos_SetVoltage.vi"("commit"=TRUE, "pHandle"=w1369, "error in"=w1370, "value"=w1364, "voltageName"=w1368, "dll path in"=w1372) -> ("error out"=w1375:errorcluster, "dll path out"=w1376:path)  [unwired: 3 in]
        }
      }
      frame "setsgl" {
        n663 = Dequeue Element(queue=w1416) -> ()  [unwired: 2 in, 4 out]
        n664 = Match Pattern(string=w1412, regular expression=":") -> (before substring=w1405:string, after substring=w1414:string)  [unwired: 1 in, 2 out]
        n665 = Equal?(x=w1414, y="wait") -> ()  [unwired: 1 out]
        n666 = Match Pattern(string=w1405, regular expression=":") -> (before substring=w1379:string, after substring=w1404:string)  [unwired: 1 in, 2 out]
        n667 = Fract/Exp String To Number(string=w1404) -> (number=w1403:dbl)  [unwired: 3 in, 1 out]
        n668 = call "SL2_AD_DLL_Phoibos_GetVoltageRange.vi"("voltage_name"=w1379, "pHandle"=w1400, "dll path in"=w1402) -> ("error out"=w1409:errorcluster, "min"=w1407:dbl, "max"=w1408:dbl, "dll path out"=w1410:path)  [unwired: 3 in]
        n669 = In Range and Coerce(upper limit=w1408, x=w1403, lower limit=w1407) -> (coerced(x)=w1398:dbl)  [unwired: 1 out]
        n670 = call "SL2_AD_DLL_Phoibos_SetVoltage.vi"("commit"=TRUE, "pHandle"=w1400, "error in"=w1409, "value"=w1398, "voltageName"=w1379, "dll path in"=w1410) -> ("error out"=w1399:errorcluster, "dll path out"=w1401:path)  [unwired: 3 in]
        n671 = while {
          tunnel: w1401 -> [w1432]
          tunnel: w1400 -> [w1426]
          tunnel: w1379 -> [w1431]
          tunnel: w1399 -> [w1430]
          tunnel: w1398 -> [w1429]
          tunnel: [w1426] -> w1380
          tunnel: [w1425] -> w1382
          tunnel: [w1424] -> w1384
          stop <- w1427 stop-if-true
          n672 = call "SL2_AD_DLL_Phoibos_GetVoltage.vi"("error in"=w1430, "voltage_name"=w1431, "pHandle"=w1426, "dll path in"=w1432) -> ("error out"=w1424:errorcluster, "value"=w1428:dbl, "dll path out"=w1425:path)  [unwired: 3 in]
          n673 = Equal?(x=w1429, y=w1428) -> (x = y?=w1427:bool)
        }
        n674 = for {
          tunnel: w1380 -> [w1423]
          tunnel: [w1421] -> w1385 mode=indexing
          tunnel: [w1420] -> w1381
          shift-right: [w1419] -> w1383
          shift-left: w1384 -> [w1422]
          tunnel: w1382 -> [w1418]
          tunnel: w1378 -> [w1417] mode=indexing
          n675 = call "SL2_AD_DLL_Phoibos_GetVoltage.vi"("error in"=w1422, "voltage_name"=w1417, "pHandle"=w1423, "dll path in"=w1418) -> ("error out"=w1419:errorcluster, "value"=w1421:dbl, "dll path out"=w1420:path)  [unwired: 3 in]
        }
        n676 = Index Array(array=w1385) -> (element #1=w1386:dbl, element #2=w1387:dbl, element #3=w1388:dbl, element #4=w1389:dbl, element #5=w1390:dbl, element #6=w1394:dbl, element #7=w1391:dbl, element #8=w1392:dbl, element #9=w1393:dbl, element #10=w1377:dbl)  [unwired: 10 in]
        n677 = local write "phoib_I_1"(w1386) -> ()
        n678 = local write "phoib_I_2"(w1387) -> ()
        n679 = local write "phoib_I_3"(w1388) -> ()
        n680 = local write "phoib_I_4"(w1389) -> ()
        n681 = local write "phoib_I_5"(w1390) -> ()
        n682 = local write "phoib_I_6"(w1394) -> ()
        n683 = local write "phoib_I_7"(w1391) -> ()
        n684 = local write "phoib_I_8"(w1392) -> ()
        n685 = local write "phoib_I_9"(w1393) -> ()
        n686 = local write "phoib_I_10"(w1377) -> ()
        n687 = Send Notification(notification=TRUE, notifier=w1396, error in (no error)=w1383) -> (error out=w1397:errorcluster)  [unwired: 1 out]
      }
      frame "standby" {
        w1439 = T2 0 items=["Off"=-1, "Standby"=0, "On"=1] ("state")
        n688 = Dequeue Element(queue=w1433) -> ()  [unwired: 2 in, 4 out]
        n689 = call "SL2_AD_DLL_Phoibos_SetDeviceState.vi"("pHandle_in"=w1434, "error in"=w1437, "state"=w1439, "dev_type"=DEF_dev_type."devA (analyzer)", "dll_path"=w1438) -> ("error out"=w1435:errorcluster, "path out"=w1436:path)  [unwired: 2 in]
      }
      frame "release" {
        n690 = Dequeue Element(queue=w1451) -> (queue out=w1441:refnum<queue>)  [unwired: 2 in, 3 out]
        n691 = flat-sequence {
          tunnel: w1450 -> [w1452]
          tunnel: w1446 -> [w1453]
          tunnel: [w1456] -> w1445
          tunnel: [w1455] -> w1444
          tunnel: [u32 0] -> w1443
          tunnel: [w1458] -> w1447
          tunnel: [w1459] -> w1448
          tunnel: [w1460] -> w1449
          tunnel: w1445 -> [w1460]
          tunnel: w1444 -> [w1459]
          tunnel: w1443 -> [w1458]
          frame #0 {
            n692 = call "SL2_AD_DLL_Phoibos_Shutdown.vi"("pHandle"=w1453, "dll path in"=w1452) -> ("error out"=w1455:errorcluster, "dll path out"=w1456:path)  [unwired: 4 in]
          }
          frame #1 {
            n693 = local write "phoib_con?"(FALSE ("phoib_con?")) -> ()
          }
        }
        n694 = Enqueue Element(queue=w1441, element="suspend") -> ()  [unwired: 2 in, 3 out]
      }
      frame "close" {
        n695 = Release Queue(queue=w1465) -> ()  [unwired: 2 in, 3 out]
      }
      frame "suspend" {
        n696 = Dequeue Element(queue=w1470) -> ()  [unwired: 2 in, 4 out]
      }
      frame "init" {
        n697 = Dequeue Element(queue=w1475) -> ()  [unwired: 2 in, 4 out]
        n698 = flat-sequence {
          tunnel: [w1482] -> w1473
          tunnel: [w1478] -> w1472
          tunnel: [w1477] -> w1471
          tunnel: [w1490] -> w1474
          tunnel: w1473 -> [w1490]
          frame #0 {
            n699 = local write "phoib_con?"(FALSE ("phoib_con?")) -> ()
          }
          frame #1 {
            w1481 = DEF_dev_type."devA (analyzer)" ("dev_type")
            n700 = call "GetSL2AD_VI_dllPath.vi"() -> ("error"=w1485:errorcluster, "Path"=w1486:path)  [unwired: 9 in, 1 out]
            n701 = call "SL2_AD_DLL_List_Devices.vi"("error in"=w1485, "dev_type"=w1481, "dll path in"=w1486) -> ("error out"=w1479:errorcluster, "devices"=w1488:string[], "dll path out"=w1480:path)  [unwired: 2 in]
            n702 = Index Array(array=w1488) -> (element=w1487:string)  [unwired: 1 in]
            n703 = call "SL2_AD_DLL_Phoibos_Initialize.vi"("error in"=w1479, "analyzerId"=w1487, "dll_path"=w1480) -> ("error out"=w1483:errorcluster, "pHandle"=w1482:u32, "path out"=w1484:path)  [unwired: 2 in]
            n704 = call "SL2_AD_DLL_Phoibos_ListDeviceModes.vi"("dll path in"=w1484, "dev_type"=w1481, "pHandle"=w1482, "error in"=w1483) -> ("dll path out"=w1478:path, "error out"=w1477:errorcluster)  [unwired: 1 in, 2 out]
          }
          frame #2 {
            n705 = local write "phoib_con?"(TRUE ("phoib_con?")) -> ()
          }
        }
      }
    }
    "phoib_error" <- w1295
  }
  n706 = while {
    tunnel: w1 -> [w1500]
    tunnel: w5 -> [w1494]
    shift-right: [w1493] -> _
    shift-left: 0 -> [w1492]
    stop <- w1491 stop-if-true
    # "temp"
    n707 = Preview Queue Element(queue=w1500, timeout in ms (-1)=w1492) -> (queue out=w1495:refnum<queue>, element=w1499:string)  [unwired: 1 in, 2 out]
    n708 = Match Pattern(string=w1499, regular expression=":") -> (before substring=w1498:string, after substring=w1497:string)  [unwired: 1 in, 2 out]
    n709 = case shown="\"ramp\"" w1498 {
      tunnel: w1497 -> [w1506 _ _ _ _]
      tunnel: w1495 -> [w1501 w1526 w1527 _ w1540]
      tunnel: w1494 -> [w1502 _ _ _ _]
      tunnel: [_ _ _ _ -1] -> w1493
      tunnel: [_ TRUE _ _ _] -> w1491
      frame "ramp" {
        n710 = Dequeue Element(queue=w1501) -> ()  [unwired: 2 in, 4 out]
        n711 = Match Pattern(string=w1506, regular expression=":") -> (before substring=w1505:string, after substring=w1509:string)  [unwired: 1 in, 2 out]
        n712 = Equal?(x=w1509, y="wait") -> (x = y?=w1503:bool)
        n713 = Scan From String(input string=w1505) -> (output 1=w1504:dbl)  [unwired: 4 in, 3 out]
        n714 = flat-sequence {
          tunnel: w1504 -> [w1511]
          tunnel: w1503 -> [w1513]
          tunnel: w1502 -> [w1523]
          frame #0 {
            n715 = local read "LS310  EPICS SP"() -> (w1510:string)
            n716 = call-poly <userlib>:"CaLabPut.vi"("Value"=w1511, "PV Name"=w1510) -> ()  [unwired: 6 in, 4 out]
          }
          frame #1 {
            n717 = Wait (ms)(milliseconds to wait=500) -> ()  [unwired: 1 out]
          }
          frame #2 {
            n718 = case shown="True" w1513 {
              frame False {
              }
              frame True {
                n719 = while {
                  stop <- w1519 stop-if-true
                  n720 = local read "Status EPICS chanel"() -> (w1521:string)
                  n721 = Wait (ms)(milliseconds to wait=500) -> ()  [unwired: 1 out]
                  n722 = call-poly <userlib>:"CaLabGet.vi"("PV Name"=w1521) -> ("1rst Value (string)"=w1522:string)  [unwired: 8 in, 6 out]
                  n723 = Equal?(x=w1522, y="Inside Range") -> (x = y?=w1519:bool)
                  n724 = local read "LS310  EPICS chanel A"() -> (w1515:string)
                  n725 = local read "LS310  EPICS chanel B"() -> (w1514:string)
                  n726 = call-poly <userlib>:"CaLabGet.vi"("PV Name"=w1515) -> ("1rst Value (number)"=w1516:dbl)  [unwired: 8 in, 6 out]
                  n727 = call-poly <userlib>:"CaLabGet.vi"("PV Name"=w1514) -> ("1rst Value (number)"=w1517:dbl)  [unwired: 8 in, 6 out]
                  n728 = local write "TB"(w1517) -> ()
                  n729 = local write "TA"(w1516) -> ()
                }
              }
            }
          }
          frame #3 {
            n730 = Send Notification(notification=TRUE, notifier=w1523) -> ()  [unwired: 1 in, 2 out]
          }
        }
      }
      frame "close" {
        n731 = Release Queue(queue=w1526) -> ()  [unwired: 2 in, 3 out]
      }
      frame "init" {
        n732 = Dequeue Element(queue=w1527) -> ()  [unwired: 2 in, 4 out]
      }
      frame "idle", Default {
        n733 = local read "LS310  EPICS chanel A"() -> (w1538:string)
        n734 = local read "LS310  EPICS chanel B"() -> (w1537:string)
        n735 = local read "LS310  EPICS SP"() -> (w1528:string)
        n736 = local read "Status EPICS chanel"() -> (w1536:string)
        n737 = local read "LS310  EPICS Heater"() -> (w1535:string)
        n738 = call-poly <userlib>:"CaLabGet.vi"("PV Name"=w1538) -> ("1rst Value (number)"=→"TA":dbl)  [unwired: 8 in, 6 out]
        n739 = call-poly <userlib>:"CaLabGet.vi"("PV Name"=w1537) -> ("1rst Value (number)"=→"TB":dbl)  [unwired: 8 in, 6 out]
        n740 = call-poly <userlib>:"CaLabGet.vi"("PV Name"=w1528) -> ("1rst Value (number)"=→"Readback":dbl)  [unwired: 8 in, 6 out]
        n741 = call-poly <userlib>:"CaLabGet.vi"("PV Name"=w1536) -> ("1rst Value (string)"=w1532:string)  [unwired: 8 in, 6 out]
        n742 = call-poly <userlib>:"CaLabGet.vi"("PV Name"=w1535) -> ()  [unwired: 8 in, 7 out]
        n743 = Equal?(x=w1532, y="Inside Range") -> (x = y?=→"In Range":bool)
      }
      frame "suspend" {
        n744 = Dequeue Element(queue=w1540) -> ()  [unwired: 2 in, 4 out]
      }
    }
  }
